vi "MC_10_19a_JW6.vi"() -> ()   [LabVIEW 2011]
uses:
  <vilib>/Utility/file.llb/Read From Spreadsheet File (string).vi
  <vilib>/Utility/inputDevices.llb/keyboardAcquire.vi
  <vilib>/Utility/file.llb/Write To Spreadsheet File (DBL).vi
  <vilib>/Utility/file.llb/Write To Spreadsheet File (string).vi
  <vilib>/regexp/Match Regular Expression.xnode
panel:
  out "Current \nRecord":string[](array[string])
  out "Transformer \nHeaders":string[](array[string])
  out "Current Device ID":string
  out "Column":string
  out "Row":string
  out "Date Recorded":string="Date Recorded"
  out "Concentration Recorded":string
  out "Solvent Recorded":string
  out "Method Recorded":string
  in  "?":T1(tab)
  out "Material Recorded":string
  in  "Treatment Concentration (mM):":dbl=30.0
  in  "Surface Treatment:":string
  in  "# Drops:":dbl=inf
  in  "Solution Temp (C):":dbl=55.0
  in  "Relative Humidity (%):":dbl=nan
  in  "Room Temp (F):":dbl=nan
  in  "Time (s):":dbl=80.0
  out "Accel (RPM/s):":dbl
  in  "RPM:":dbl=1000.0
  in  "Wait Time (s):":dbl=10.0
  in  "Sample #:":dbl=1.0
  in  "Fabricator:":string="Jeremy"
  in  "Data File":path
  out "Data Folder":path
  in  "Image Folder":path
  out "Image File":path
  in  "Ramp (s):":dbl=3.0
  out "Mobility":dbl format="%#_4e"
  out "Length":dbl
  out "Width":dbl
  out "Dielectric (d)":dbl
  out "XY Graph":cluster{dbl[], dbl[]}[](graph)
  in  "NumPts":dbl=5.0
  in  "Cancel Button":bool
  in  "Next Button":bool
  in  "Previous Button":bool
  in  "Up Button":bool
  in  "Down Button":bool
  out "Data Name":string
  in  "Save Changes?":bool
  in  "New Dielectric":dbl
  in  "New Length":dbl
  in  "New Width":dbl
  out "New Mobility":dbl format="%#_4e"
  in  "Slide":dbl(slide) step=1.0 scale=-14.3..84.0 scale format="%#_1p"
  in  "Blank Button":bool
  in  "Zoom":i16(slide)=-3 scale=-5.0..5.0
  out "Image Out 2":T2(plugin-control)
  out "Image Out":T2(plugin-control)
  in  "Magnification":u16(ring) items=["5x", "10x", "20x", "50x", "80x"]
  out "Total Width":dbl
  out "Distances":dbl[](array[numeric])
  in  "Undo Button":bool
  in  "Remove Button":bool
  out "Recorded Mobility":dbl format="%#_4e"
  out "Index 3":string
  out "Image Name":string
  in  "Export":bool
  out "Threshold V":dbl
  out "New Vt":dbl
  in  "Manual":bool
  out "XY Graph 2":cluster{dbl[], dbl[]}[](graph)
  in  "Next Button 2":bool
  in  "Previous Button 2":bool
  in  "Slide 2":dbl(slide) step=1.0 scale=-1.0..82.0 scale format="%#_1p"
  out "S.T.S.":dbl
  out "New S.T.S.":dbl
  in  "NumPts 2":dbl=5.0
  out "Vt recorded":dbl
  out "STS recorded":dbl
  out "On/Off":dbl format="%#_3e"
  in  "Save Changes? 2":bool
  in  "Save Changes? 3":bool
  out "String":string
  in  "No Image":path=path "C:/Program Files/Mega Awesome/Image Not Found.png"
  in  "Project":path=path "C:/Program Files/Mega Awesome/DeviceData.opj"
  out "Index 2":dbl
  out "Array 8":dbl[](array[numeric])
  out "Array 7":dbl[](array[numeric])
  out "ROI Descriptor out":T3 {"Contours"."Type" items=["No Selection", "Point", "Line", "Rectangle", "Oval", "Polygon", "Freehand Region", "Annulus", "Unused2", "Unused3", "Broken Line", "Freehand Line", "Rotated Rectangle"]}
  out "ROI Descriptor":T3 {"Contours"."Type" items=["No Selection", "Point", "Line", "Rectangle", "Oval", "Polygon", "Freehand Region", "Annulus", "Unused2", "Unused3", "Broken Line", "Freehand Line", "Rotated Rectangle"]}
  out "Numeric 3":dbl
  out "Array 6":dbl[][](array[numeric])
  out "Cluster":T4
  out "Array 5":dbl[](array[numeric])
  out "Array 4":dbl[](array[numeric])
  out "Array 3":dbl[](array[numeric])
  out "Numeric 2":dbl
  out "Numeric":dbl
  out "Array 2":dbl[](array[numeric])
  out "Array":dbl[](array[numeric])
  out "Index":dbl
  out "Table Control 2":string[][](table)
  out "Table Control":string[][](table)
  in  "Row Start":dbl=20.0
  # "Data Locations"
  # "Data Location"
  # "Image Location"
  # "Sample Properties"
  # "Recorded"
  # "Calculated"
  # "Re-Calculated"
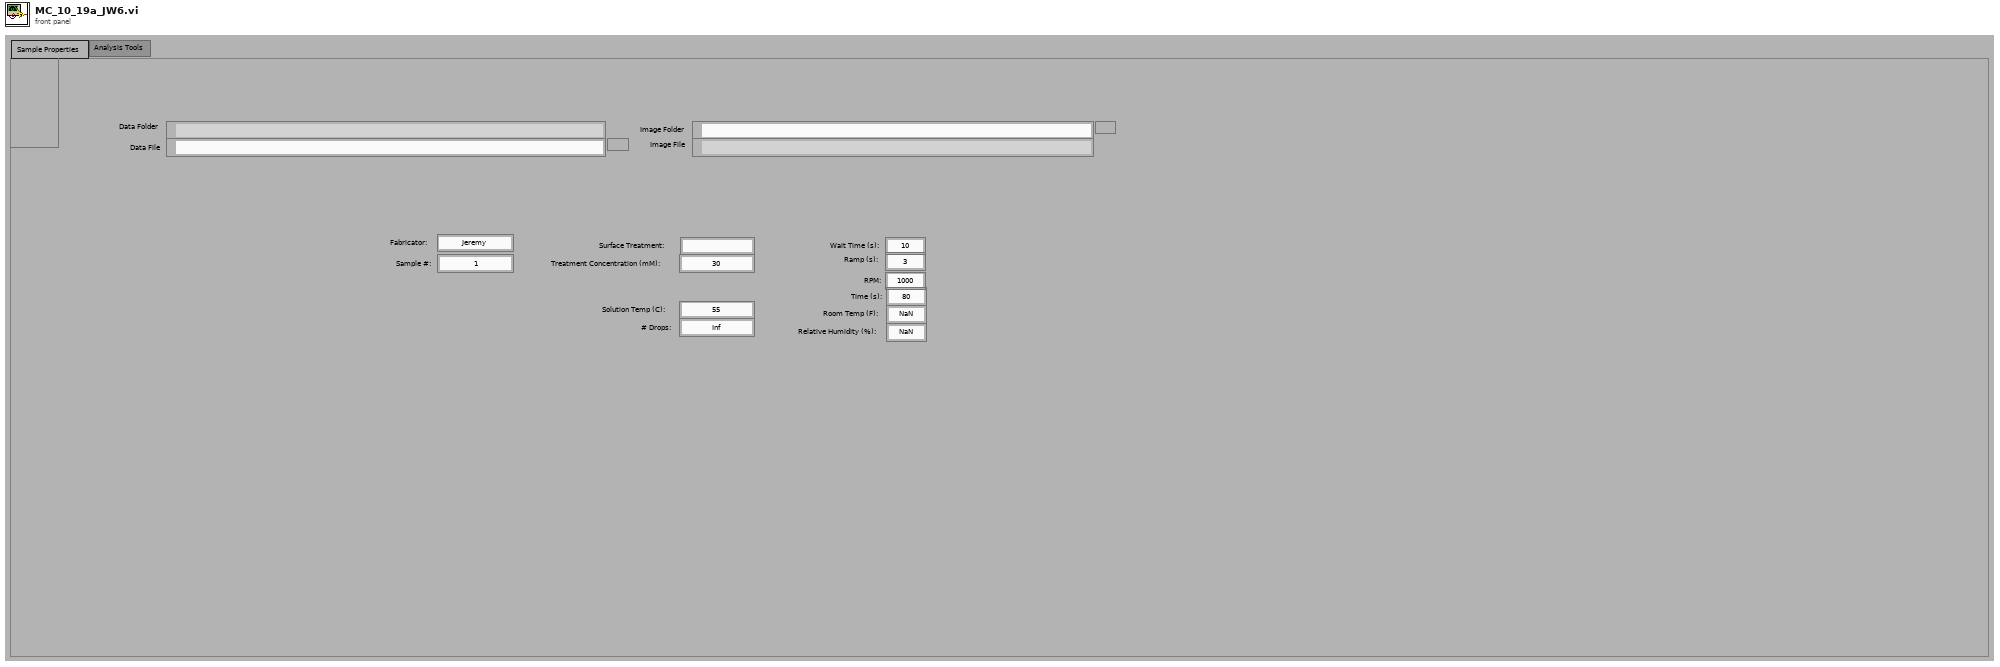
[diagram p1: front panel]
types:
  T1 = enum32{"Sample Properties", "Analysis Tools", "Current Database"}
  T2 = typedef "IMAQ Image.ctl" = refnum<image>
  T3 = typedef "ROI Descriptor" = cluster{"Global Rectangle":i32[], "Contours":cluster{"ID":enum32{"External", "Internal"}, "Type":u32, "Coordinates":i32[]}[]}
  T4 = cluster{"Numeric":dbl, "Numeric 2":dbl, "Numeric 3":dbl, "Numeric 4":dbl}
  T5 = cluster{"[0]":cluster{dbl[], dbl[]}, "[1]":cluster{dbl[], dbl[]}, "[2]":cluster{dbl[], dbl[]}, "[3]":cluster{dbl[], dbl[]}, "[4]":cluster{dbl[], dbl[]}, "[5]":cluster{dbl[], dbl[]}, "[6]":cluster{dbl[], dbl[]}, "[7]":cluster{dbl[], dbl[]}, "[8]":cluster{dbl[], dbl[]}}
  T6 = cluster{"Vt":dbl, "STS":dbl, "On/Off":dbl, "Deposition":string, "Solvent":string, "Concentration":string, "Material":string}
  T7 = cluster{"Global Rectangle":i32[], "Contours":cluster{"Contour Type":u32, "ROI Type":u32, "Points":i32[]}[]}
  T8 = typedef "LVBoundsTypeDef.ctl" = cluster{"Width":u32, "Height":u32}
  T9 = cluster{"Contour Type":u32, "ROI Type":u32, "Points":i32[]}[]
  T10 = enum16{"0", "1", "2", "3", "4", "5", "6", "7", "8", "9", "A", "B", "C", "D", "E", "F", "G", "H", "I", "J", "K", "L", "M", "N", "O", "P", "Q", "R", "S", "T", "U", "V", "W", "X", "Y", "Z", "F1", "F2", "F3", "F4", "F5", "F6", "F7", "F8", "F9", "F10", "F11", "F12", "F13", "F14", "F15", "ADD", "BACK", "BACKSLASH", "CAPITAL", "COMMA", "DECIMAL", "DELETE", "DIVIDE", "DOWN", "END", "EQUALS", "ESCAPE", "GRAVE (`)", "HOME", "INSERT", "LBRACKET", "LCONTROL", "LEFT", "L ALT", "LSHIFT", "LWIN", "MINUS", "MULTIPLY", "NEXT", "NUMLOCK", "NUMPAD_0", "NUMPAD_1", "NUMPAD_2", "NUMPAD_3", "NUMPAD_4", "NUMPAD_5", "NUMPAD_6", "NUMPAD_7", "NUMPAD_8", "NUMPAD_9", "PAUSE", "PERIOD", "PRIOR (PG UP)", "RBRACKET", "RCONTROL", "RETURN", "RIGHT", "R ALT", "RSHIFT", "RWIN", "SCROLL", "SEMICOLON", "SLASH", "SPACE", "SUBTRACT", "TAB", "UP", "ENTER (num pad)", "' (quote)"}[]
  T11 = cluster{i32[], cluster{"Contour Type":u32, "ROI Type":u32, "Points":i32[]}[]}
  T12 = enum16{"0", "1", "2", "3", "4", "5", "6", "7", "8", "9", "A", "B", "C", "D", "E", "F", "G", "H", "I", "J", "K", "L", "M", "N", "O", "P", "Q", "R", "S", "T", "U", "V", "W", "X", "Y", "Z", "F1", "F2", "F3", "F4", "F5", "F6", "F7", "F8", "F9", "F10", "F11", "F12", "F13", "F14", "F15", "ADD", "BACK", "BACKSLASH", "CAPITAL", "COMMA", "DECIMAL", "DELETE", "DIVIDE", "DOWN", "END", "EQUALS", "ESCAPE", "GRAVE (`)", "HOME", "INSERT", "LBRACKET", "LCONTROL", "LEFT", "L ALT", "LSHIFT", "LWIN", "MINUS", "MULTIPLY", "NEXT", "NUMLOCK", "NUMPAD_0", "NUMPAD_1", "NUMPAD_2", "NUMPAD_3", "NUMPAD_4", "NUMPAD_5", "NUMPAD_6", "NUMPAD_7", "NUMPAD_8", "NUMPAD_9", "PAUSE", "PERIOD", "PRIOR (PG UP)", "RBRACKET", "RCONTROL", "RETURN", "RIGHT", "R ALT", "RSHIFT", "RWIN", "SCROLL", "SEMICOLON", "SLASH", "SPACE", "SUBTRACT", "TAB", "UP", "ENTER (num pad)", "' (quote)"}
  T13 = cluster{string, sgl, bool, bool, bool, bool, bool, bool, i32}
  T14 = cluster{i32, cluster{string, sgl, bool, bool, bool, bool, bool, bool, i32}, i32, i32}
  T15 = cluster{"Contour Type":u32, "ROI Type":u32, "Points":i32[]}
  T16 = cluster{"Points[0]":i32, "Points[1]":i32, "Points[2]":i32, "Points[3]":i32, "Points[4]":i32, "Points[5]":i32, "Points[6]":i32, "Points[7]":i32, "Points[8]":i32}
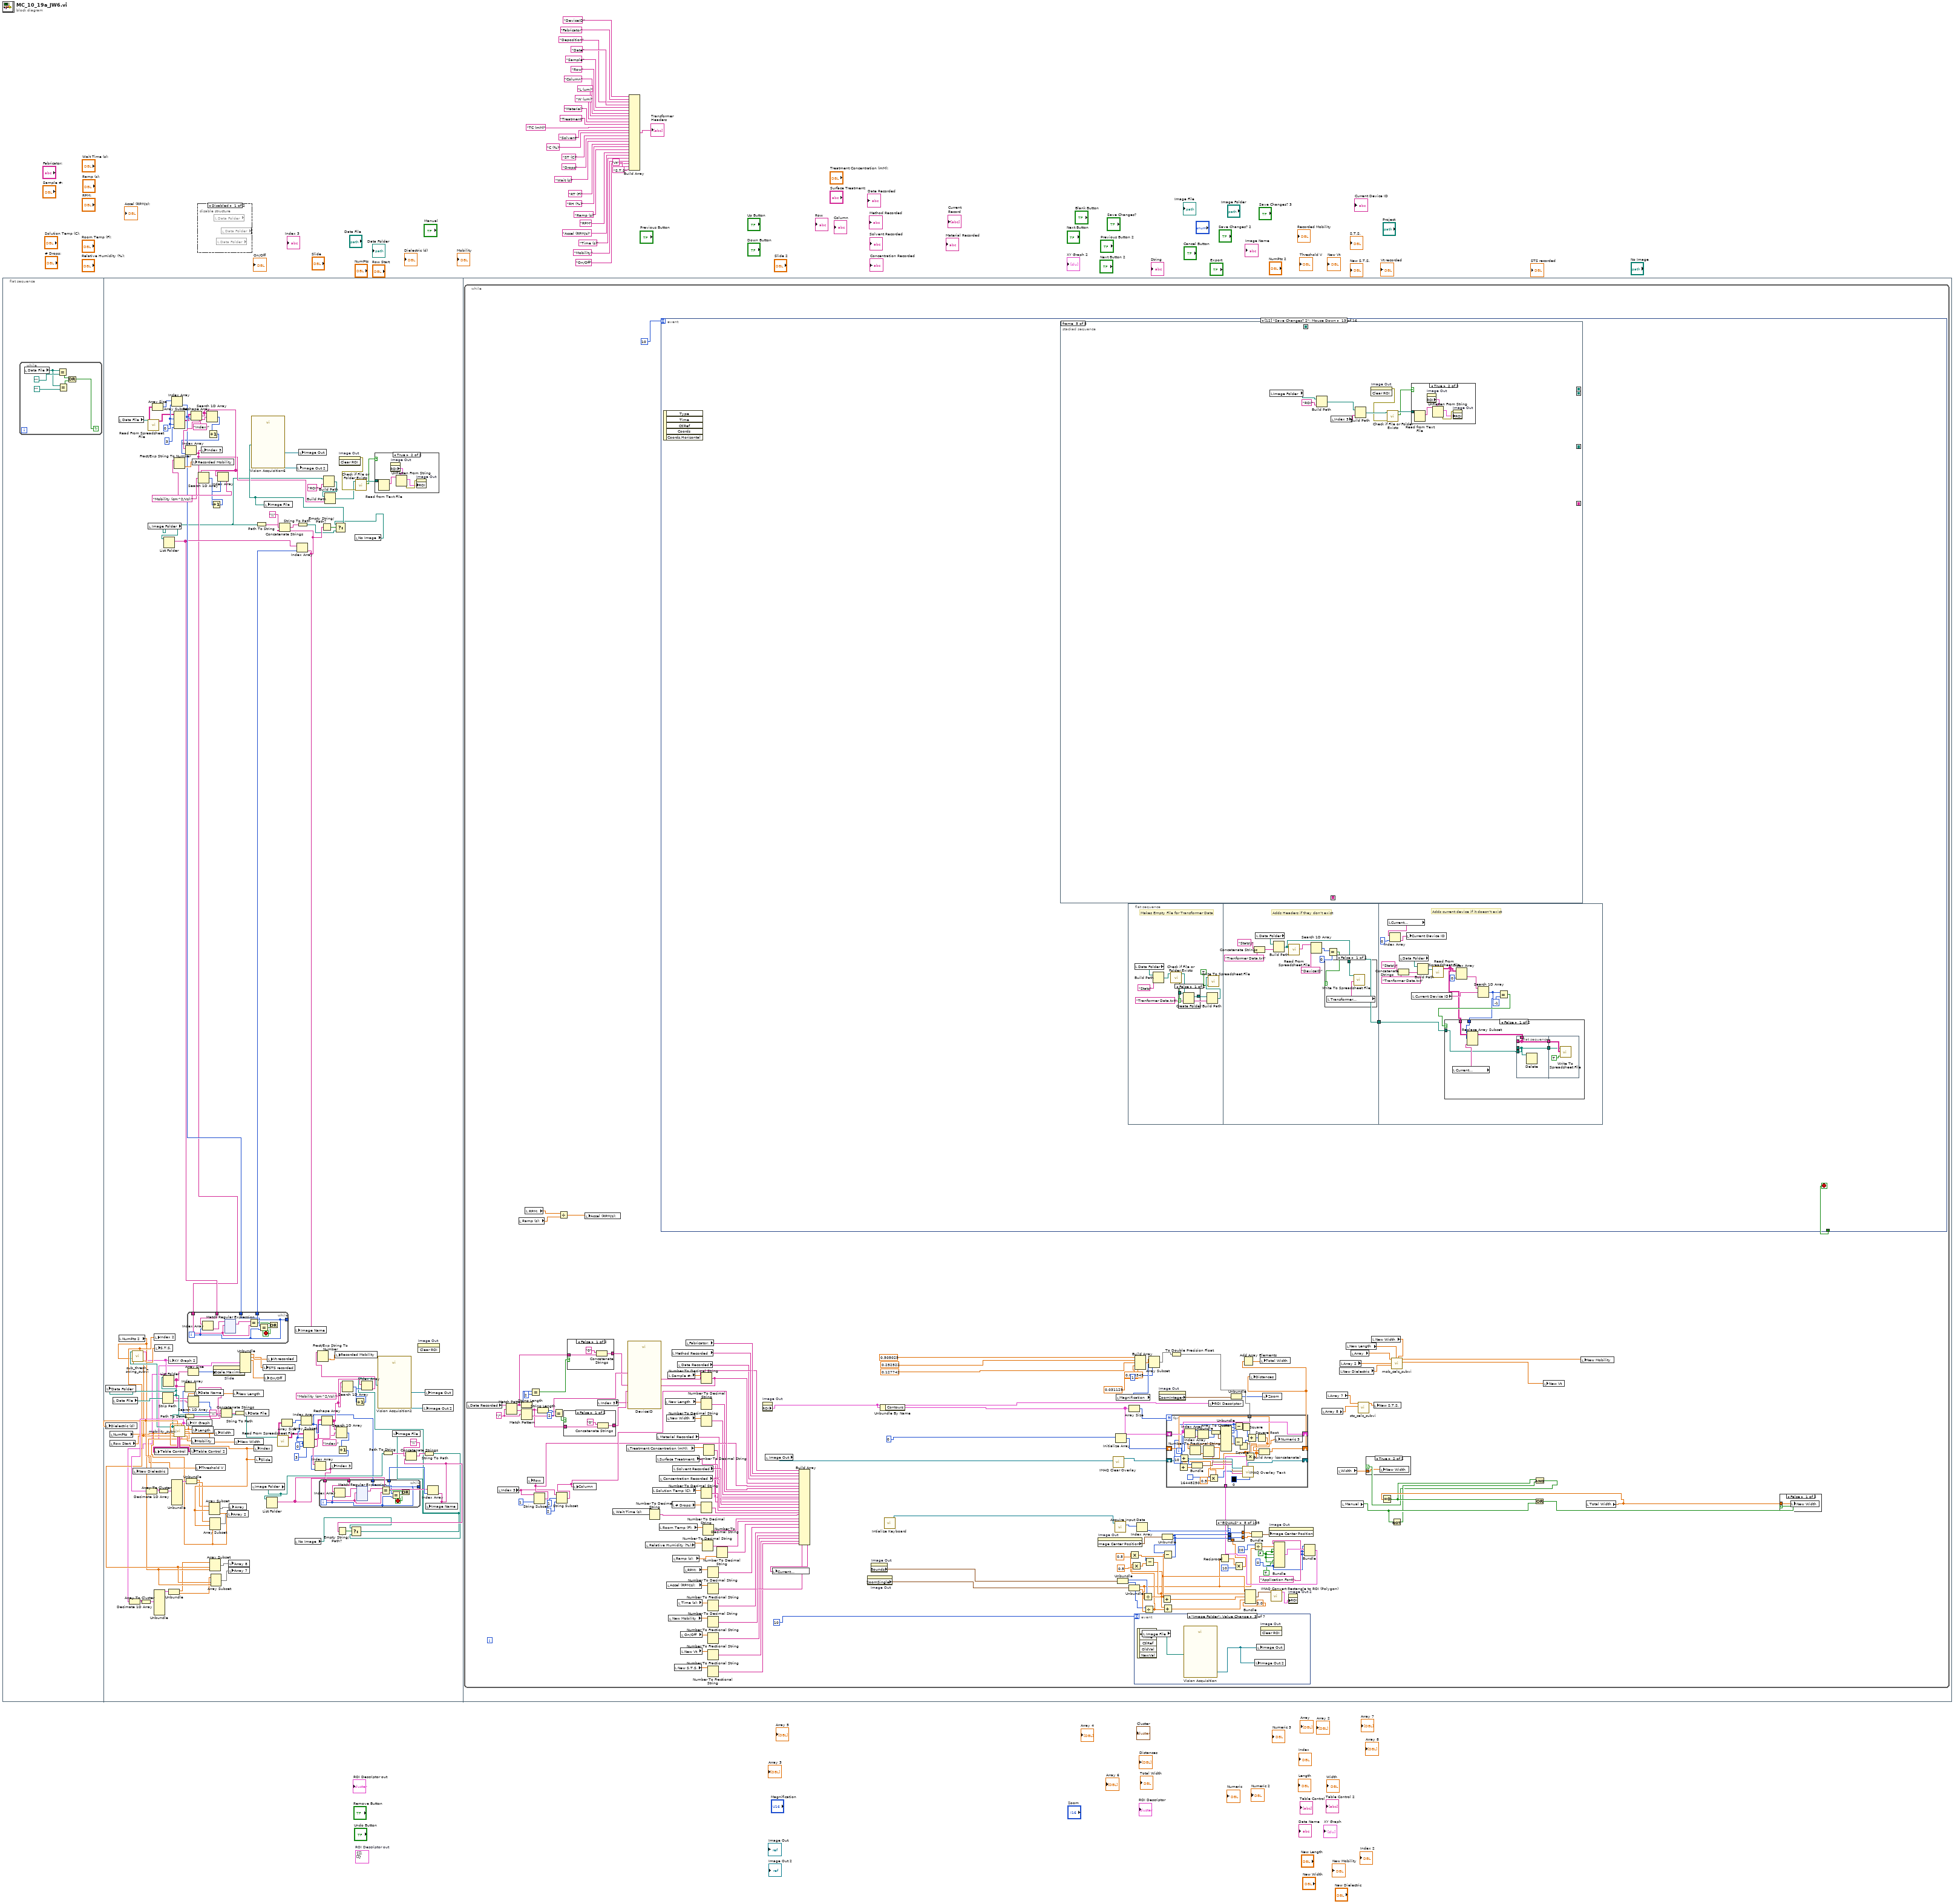
[diagram p0: block diagram]
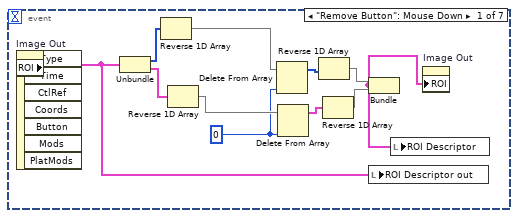
[diagram p7: hidden frame]
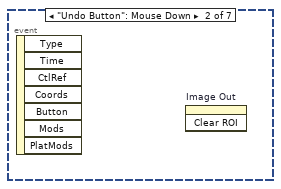
[diagram p8: hidden frame]
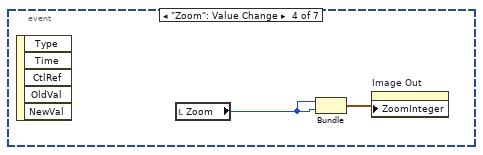
[diagram p9: hidden frame]
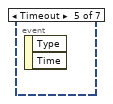
[diagram p10: hidden frame]
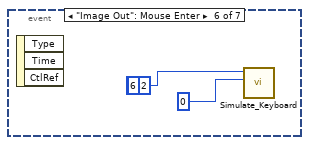
[diagram p11: hidden frame]
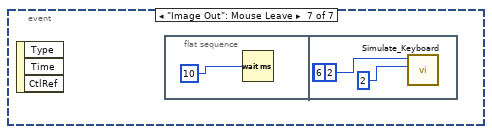
[diagram p12: hidden frame]
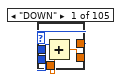
[diagram p13: hidden frame]
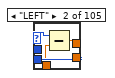
[diagram p14: hidden frame]
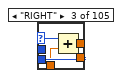
[diagram p15: hidden frame]
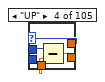
[diagram p16: hidden frame]
diagram:
  (unwired) T3 {"Global Rectangle"=[], "Contours"=[]}  # ROI Descriptor out
  n1 = flat-sequence {
    frame #0 {
      n2 = while {
        stop <- w29 continue-if-true
        n3 = local read "Data File"() -> (w31:path)
        n4 = Equal?(x=w31, y=path "") -> (x = y?=w33:bool)
        n5 = Equal?(x=w31, y=path "") -> (x = y?=w32:bool)
        n6 = Or(x=w33, y=w32) -> (x .or. y?=w29:bool)
      }
    }
    frame #1 {
      w95 = 0
      w125 = 0
      n7 = local read "NumPts"() -> (w70:dbl)
      n8 = local read "Row Start"() -> (w69:dbl)
      n9 = local read "Data File"() -> (w99:path)
      n10 = local read "Data File"() -> (w120:path)
      n11 = local read "NumPts 2"() -> (w64:dbl)
      n12 = call-poly <vilib>:"Read From Spreadsheet File.vi"("file path (dialog if empty)"=w120) -> ("all rows"=w123:string[][])  [unwired: 6 in, 4 out]
      n13 = local read "Image Folder"() -> (w35:path)
      n14 = Array Size(array=w123) -> (size(s)=w124:i32[])
      n15 = Strip Path(path=w99) -> (stripped path=w100:path, name=w81:string)
      n16 = local write "Data Folder"(w100) -> ()
      n17 = List Folder(path=w100) -> (filenames=w89:string[])  [unwired: 3 in, 3 out]
      n18 = List Folder(path=w35) -> (filenames=w129:string[])  [unwired: 3 in, 3 out]
      n19 = Index Array(array=w124, index=w125) -> (element=w131:i32)
      n20 = Array Subset(array=w123, index (row)=w125, index (col)=w125, length (col)=3) -> (w122:string[][])  [unwired: 1 in]
      n21 = Path To String(path=w100) -> (string=w80:string)
      n22 = Array Size(array=w89) -> (size(s)=w90:i32)
      n23 = Search 1D Array(1D array=w89, element=w81) -> (index of element=w88:i32)  [unwired: 1 in]
      n24 = Index Array(array=w89, index=w88) -> (element=w87:string)
      n25 = Reshape Array(w122, w131) -> (w141:string[])
      n26 = local write "Data Name"(w87) -> ()
      n27 = Search 1D Array(1D array=w141, element="Mobility (cm^2/Vs):") -> (index of element=w136:i32)  [unwired: 1 in]
      n28 = Search 1D Array(1D array=w141, element="Index:") -> (index of element=w128:i32)  [unwired: 1 in]
      n29 = Increment(x=w128) -> (x+1=w127:i32)
      n30 = Index Array(array=w141, index=w127) -> (element=w36:string)
      n31 = while {
        tunnel: w129 -> [w274]
        tunnel: w36 -> [w272]
        tunnel: [w271] -> _
        tunnel: [w271] -> w130
        tunnel: w131 -> [w270]
        i -> [w271]
        stop <- w267 stop-if-true
        n32 = Index Array(array=w274, index=w271) -> (element=w275:string)
        n33 = xnode "Match Regular Expression"("input string"=w275, "regular expression"=w272) -> ("whole match"=w273:string)  [unwired: 4 in, 4 out]
        n34 = Equal?(x=w273, y=w272) -> (x = y?=w269:bool)
        n35 = Equal?(x=w270, y=w271) -> (x = y?=w268:bool)
        n36 = Or(x=w269, y=w268) -> (x .or. y?=w267:bool)
      }
      n37 = local write "Index 3"(w36) -> ()
      n38 = Increment(x=w136) -> (x+1=w137:i32)
      n39 = property on="Slide" class="Slide (strict)"("Scale.Maximum"=w90) -> ()  [unwired: 2 in, 2 out]
      n40 = Index Array(array=w141, index=w137) -> (element=w139:string)
      n41 = Fract/Exp String To Number(string=w139) -> (number=w140:dbl)  [unwired: 3 in, 1 out]
      n42 = local write "Recorded Mobility"(w140) -> ()
      n43 = Concatenate Strings(w80, "\\", w87) -> (w82:string)
      n44 = String To Path(string=w82) -> (path=w71:path)
      n45 = call "sub_thresh_swing_subvi.vi"("Path"=w71, "NumPts"=w64, "Row Start"=w69) -> ("Index"=w65:dbl, "XY Graph"=w60:cluster{dbl[], dbl[]}[], "Sub Threshold Swing"=w72:dbl)  [unwired: 8 in, 2 out]
      n46 = Decimate 1D Array(w60) -> (w61:cluster{dbl[], dbl[]}[])  [unwired: 1 out]
      n47 = Array To Cluster(array=w61) -> (cluster=w63:T5)
      n48 = local write "Index 2"(w65) -> ()
      n49 = Unbundle(w63) -> ("[0]"=w62:cluster{dbl[], dbl[]})  [unwired: 8 out]
      n50 = local write "S.T.S."(w72) -> ()
      n51 = local write "XY Graph 2"(w60) -> ()
      n52 = Unbundle(w62) -> (w58:dbl[], w57:dbl[])
      n53 = call "mobility_subvi.vi"("Path"=w71, "NumPts"=w70, "Row Start"=w69) -> ("Dielectric (d)"=w76:dbl, "Index"=w77:dbl, "XY Graph"=w119:cluster{dbl[], dbl[]}[], "Length"=w75:dbl, "Vt"=w73:dbl, "Width"=w74:dbl, "Table Control"=w84:string[][], "Table Control 2"=w85:string[][], "Recorded"=w54:T6, "Mobility"=w86:dbl)  [unwired: 2 in, 1 out]
      n54 = local write "Dielectric (d)"(w76) -> ()
      n55 = local write "New Dielectric"(w76) -> ()
      n56 = Decimate 1D Array(w119) -> (w118:cluster{dbl[], dbl[]}[])  [unwired: 1 out]
      n57 = local write "Table Control"(w84) -> ()
      n58 = Array To Cluster(array=w118) -> (cluster=w116:T5)
      n59 = Unbundle(w116) -> ("[0]"=w117:cluster{dbl[], dbl[]})  [unwired: 8 out]
      n60 = Unbundle(w117) -> (w59:dbl[], w66:dbl[])
      n61 = local write "XY Graph"(w119) -> ()
      n62 = local write "Table Control 2"(w85) -> ()
      n63 = local write "Mobility"(w86) -> ()
      n64 = local write "Length"(w75) -> ()
      n65 = local write "Threshold V"(w73) -> ()
      n66 = Array Subset(array=w59, index=w77, length=w70) -> (w78:dbl[])
      n67 = Array Subset(array=w66, index=w77, length=w70) -> (w79:dbl[])
      n68 = Array Subset(array=w58, index=w65, length=w64) -> (w68:dbl[])
      n69 = Array Subset(array=w57, index=w65, length=w64) -> (w67:dbl[])
      n70 = local write "Width"(w74) -> ()
      n71 = local write "Array 2"(w79) -> ()
      n72 = local write "Array 8"(w68) -> ()
      n73 = local write "Array 7"(w67) -> ()
      n74 = local write "Array"(w78) -> ()
      n75 = local write "New Length"(w75) -> ()
      n76 = local write "New Width"(w74) -> ()
      n77 = Unbundle(w54) -> ("Vt"=w56:dbl, "STS"=w55:dbl, "On/Off"=w53:dbl)  [unwired: 4 out]
      n78 = local write "Data File"(w71) -> ()
      n79 = local read "Image Folder"() -> (w106:path)
      n80 = local write "Index"(w77) -> ()
      n81 = local write "Slide"(w77) -> ()
      n82 = Path To String(path=w35) -> (string=w133:string)
      n83 = local write "STS recorded"(w55) -> ()
      n84 = local write "On/Off"(w53) -> ()
      n85 = List Folder(path=w106) -> (filenames=w102:string[])  [unwired: 3 in, 3 out]
      n86 = local write "Vt recorded"(w56) -> ()
      n87 = call-poly <vilib>:"Read From Spreadsheet File.vi"("file path (dialog if empty)"=w71) -> ("all rows"=w93:string[][])  [unwired: 6 in, 4 out]
      n88 = Array Size(array=w93) -> (size(s)=w94:i32[])
      n89 = local read "No Image"() -> (w44:path)
      n90 = Index Array(array=w129, index=w130) -> (element=w52:string)
      n91 = Concatenate Strings(w133, "\\", w52) -> (w134:string)
      n92 = local write "Image Name"(w52) -> ()
      n93 = String To Path(string=w134) -> (path=w50:path)
      n94 = Index Array(array=w94, index=w95) -> (element=w105:i32)
      n95 = Array Subset(array=w93, index (row)=w95, index (col)=w95, length (col)=3) -> (w92:string[][])  [unwired: 1 in]
      n96 = Empty String/Path?(string/path=w52) -> (empty?=w51:bool)
      n97 = Reshape Array(w92, w105) -> (w115:string[])
      n98 = Build Path(base path=w35, name or relative path="ROI") -> (appended path=w38:path)
      n99 = Build Path(base path=w38, name or relative path=w36) -> (appended path=w37:path)
      n100 = Search 1D Array(1D array=w115, element="Index:") -> (index of element=w98:i32)  [unwired: 1 in]
      n101 = Increment(x=w98) -> (x+1=w97:i32)
      n102 = Index Array(array=w115, index=w97) -> (element=w103:string)
      n103 = while {
        tunnel: w102 -> [w154]
        tunnel: w103 -> [w152]
        tunnel: [w151] -> _
        tunnel: [w151] -> w104
        tunnel: w105 -> [w150]
        i -> [w151]
        stop <- w147 stop-if-true
        n104 = Index Array(array=w154, index=w151) -> (element=w155:string)
        n105 = xnode "Match Regular Expression"("input string"=w155, "regular expression"=w152) -> ("whole match"=w153:string)  [unwired: 4 in, 4 out]
        n106 = Equal?(x=w153, y=w152) -> (x = y?=w149:bool)
        n107 = Equal?(x=w150, y=w151) -> (x = y?=w148:bool)
        n108 = Or(x=w149, y=w148) -> (x .or. y?=w147:bool)
      }
      n109 = local write "Index 3"(w103) -> ()
      n110 = invoke on="Image Out" class="ImageControl" method="Clear ROI"() -> (error out=w42:errorcluster)  [unwired: 3 in, 2 out]
      n111 = Search 1D Array(1D array=w115, element="Mobility (cm^2/Vs):") -> (index of element=w110:i32)  [unwired: 1 in]
      n112 = local read "No Image"() -> (w43:path)
      n113 = Select(t=w43, s=w51, f=w50) -> (s? t:f=w49:path)
      n114 = call "Vision Acquisition6"("Image Path"=w49) -> ("Image Out"=w132:T2)  [unwired: 25 in, 1 out]
      n115 = local write "Image File"(w49) -> ()
      n116 = local write "Image Out 2"(w132) -> ()
      n117 = local write "Image Out"(w132) -> ()
      n118 = Increment(x=w110) -> (x+1=w111:i32)
      n119 = call <vilib>:"Check if File or Folder Exists.vi"("error in (no error)"=w42, "path"=w37) -> ("file or folder exists?"=w40:bool, "dup path"=w41:path)  [unwired: 7 in, 1 out]
      n120 = Index Array(array=w115, index=w111) -> (element=w113:string)
      n121 = Fract/Exp String To Number(string=w113) -> (number=w114:dbl)  [unwired: 3 in, 1 out]
      n122 = local write "Recorded Mobility"(w114) -> ()
      n123 = case shown="True" w40 {
        tunnel: w41 -> [_ w142]
        frame False {
        }
        frame True {
          n124 = Read from Text File(file (use dialog)=w142) -> (text=w146:string)  [unwired: 3 in, 3 out]
          n125 = property on="Image Out" class="ImageControl"() -> ("ROI"=w143:T7)  [unwired: 2 in, 2 out]
          n126 = Unflatten From String(type=w143, binary string=w146) -> (value=w144:T7, error out=w145:errorcluster)  [unwired: 3 in, 1 out]
          n127 = property on="Image Out" class="ImageControl"(error in=w145, "ROI"=w144) -> ()  [unwired: 1 in, 2 out]
        }
      }
      n128 = Path To String(path=w106) -> (string=w107:string)
      n129 = invoke on="Image Out" class="ImageControl" method="Clear ROI"() -> ()  [unwired: 3 in, 3 out]
      n130 = Index Array(array=w102, index=w104) -> (element=w47:string)
      n131 = Empty String/Path?(string/path=w47) -> (empty?=w48:bool)
      n132 = Concatenate Strings(w107, "\\", w47) -> (w108:string)
      n133 = String To Path(string=w108) -> (path=w46:path)
      n134 = Select(t=w44, s=w48, f=w46) -> (s? t:f=w45:path)
      n135 = call "Vision Acquisition2"("Image Path"=w45) -> ("Image Out"=w101:T2)  [unwired: 25 in, 1 out]
      n136 = local write "Image File"(w45) -> ()
      n137 = local write "Image Out 2"(w101) -> ()
      n138 = local write "Image Out"(w101) -> ()
      n139 = local write "Image Name"(w47) -> ()
    }
    frame #2 {
      n140 = while {
        stop <- w533 stop-if-true
        w419 = "/"
        w483 = FALSE
        w481 = 0
        n141 = local read "Date Recorded"() -> (w422:string)
        n142 = local read "Index 3"() -> (w391:string)
        n143 = Match Pattern(string=w422, regular expression=w419) -> (before substring=w413:string, after substring=w420:string)  [unwired: 1 in, 2 out]
        n144 = local read "Ramp (s):"() -> (w388:dbl)
        n145 = String Length(string=w413) -> (length=w416:i32)
        n146 = Match Pattern(string=w420, regular expression=w419) -> (before substring=w407:string, after substring=w418:string)  [unwired: 1 in, 2 out]
        n147 = local read "RPM:"() -> (w389:dbl)
        n148 = Equal?(x=w416, y=2) -> (x = y?=w414:bool)
        n149 = String Subset(string=w391, length (rest)=1) -> (substring=w447:string)  [unwired: 1 in]
        n150 = local write "Row"(w447) -> ()
        n151 = String Length(string=w407) -> (length=w409:i32)
        n152 = Equal?(x=w409, y=2) -> (x = y?=w411:bool)
        n153 = String Subset(string=w391, offset (0)=1, length (rest)=2) -> (substring=w448:string)
        n154 = Divide(x=w389, y=w388) -> (x/y=w387:dbl)
        n155 = case shown="False" w411 {
          tunnel: w407 -> [w535 w537]
          tunnel: [w534 w537] -> w408
          frame False {
            n156 = Concatenate Strings("0", w535) -> (w534:string)
          }
          frame True {
          }
        }
        n157 = case shown="False" w414 {
          tunnel: w413 -> [w539 w541]
          tunnel: [w538 w541] -> w412
          frame False {
            n158 = Concatenate Strings("0", w539) -> (w538:string)
          }
          frame True {
          }
        }
        n159 = local write "Column"(w448) -> ()
        n160 = local write "Accel (RPM/s):"(w387) -> ()
        n161 = local read "Index 3"() -> (w406:string)
        n162 = local read "Wait Time (s):"() -> (w452:dbl)
        n163 = local read "Treatment Concentration (mM):"() -> (w399:dbl)
        n164 = local read "Relative Humidity (%):"() -> (w396:dbl)
        n165 = Number To Decimal String(number=w452) -> (decimal integer string=w453:string)  [unwired: 1 in]
        n166 = local read "Solution Temp (C):"() -> (w441:dbl)
        n167 = local read "Surface Treatment:"() -> (w398:string)
        n168 = local read "Material Recorded"() -> (w394:string)
        n169 = local read "Room Temp (F):"() -> (w445:dbl)
        n170 = local read "Concentration Recorded"() -> (w401:string)
        n171 = event shown="[12] \"Save Changes? 2\": Mouse Down" {
          selector: _ -> [_ _ _ _ _ _ _ _ _ _ _ _ _ _ _ _]
          dyn-events: _ -> [_ _ _ _ _ _ _ _ _ _ _ _ _ _ _ _]
          timeout: 10 -> [_ _ _ _ _ _ _ _ _ _ _ _ _ _ _ _]
          tunnel: [_ _ _ _ _ _ _ _ _ _ _ _ _ TRUE _ TRUE] -> w533
          event Timeout {
            n172 = event-data() -> ()  [unwired: 1 in, 2 out]
          }
          event "Down Button": Mouse Down {
            w889 = 0
            n173 = event-data() -> ()  [unwired: 1 in, 7 out]
            n174 = local read "NumPts 2"() -> (w850:dbl)
            n175 = local read "NumPts"() -> (w857:dbl)
            n176 = local read "Row Start"() -> (w856:dbl)
            n177 = local read "Data File"() -> (w894:path)
            n178 = property on="Image Out" class="ImageControl"() -> (error out=w819:errorcluster, "Image Center Position"=w823:cluster{"X":u32, "Y":u32})  [unwired: 2 in, 1 out]
            n179 = Unbundle(w823) -> ("X"=w821:u32)  [unwired: 1 out]
            n180 = Strip Path(path=w894) -> (stripped path=w885:path, name=w907:string)
            n181 = local write "Data Folder"(w885) -> ()
            n182 = List Folder(path=w885) -> (filenames=w900:string[], error out=w828:errorcluster)  [unwired: 3 in, 2 out]
            n183 = Array Size(array=w900) -> (size(s)=w895:i32)
            n184 = Bundle("X"=w821, 0) -> (w822:cluster{"X":u32, i32})  [unwired: 1 in]
            n185 = Path To String(path=w885) -> (string=w908:string)
            n186 = Search 1D Array(1D array=w900, element=w907) -> (index of element=w897:i32)  [unwired: 1 in]
            n187 = property on="Image Out" class="ImageControl"(error in=w819, "Image Center Position"=w822) -> ()  [unwired: 1 in, 2 out]
            n188 = Decrement(x=w895) -> (x-1=w898:i32)
            n189 = Equal?(x=w897, y=w898) -> (x = y?=w899:bool)
            n190 = case shown="False" w899 {
              tunnel: w897 -> [w1035 _]
              tunnel: [w1034 0] -> w896
              frame False {
                n191 = Increment(x=w1035) -> (x+1=w1034:i32)
              }
              frame True {
              }
            }
            n192 = Index Array(array=w900, index=w896) -> (element=w901:string)
            n193 = local write "Data Name"(w901) -> ()
            n194 = Concatenate Strings(w908, "\\", w901) -> (w906:string)
            n195 = String To Path(string=w906) -> (path=w858:path)
            n196 = call "sub_thresh_swing_subvi.vi"("Path"=w858, "NumPts"=w850, "Row Start"=w856) -> ("Index"=w851:dbl, "XY Graph"=w846:cluster{dbl[], dbl[]}[], "Sub Threshold Swing"=w859:dbl)  [unwired: 8 in, 2 out]
            n197 = Decimate 1D Array(w846) -> (w849:cluster{dbl[], dbl[]}[])  [unwired: 1 out]
            n198 = Array To Cluster(array=w849) -> (cluster=w847:T5)
            n199 = Unbundle(w847) -> ("[0]"=w848:cluster{dbl[], dbl[]})  [unwired: 8 out]
            n200 = Unbundle(w848) -> (w845:dbl[], w844:dbl[])
            n201 = local write "S.T.S."(w859) -> ()
            n202 = local write "XY Graph 2"(w846) -> ()
            n203 = local write "Index 2"(w851) -> ()
            n204 = call "mobility_subvi.vi"("Path"=w858, "NumPts"=w857, "Row Start"=w856) -> ("Dielectric (d)"=w861:dbl, "Date Created"=w818:string, "Index"=w866:dbl, "XY Graph"=w869:cluster{dbl[], dbl[]}[], "Length"=w860:dbl, "Vt"=w862:dbl, "Width"=w834:dbl, "Table Control"=w904:string[][], "Table Control 2"=w903:string[][], "Recorded"=w843:T6, "Mobility"=w902:dbl)  [unwired: 2 in]
            n205 = local write "Dielectric (d)"(w861) -> ()
            n206 = local write "Threshold V"(w862) -> ()
            n207 = local write "New Dielectric"(w861) -> ()
            n208 = Decimate 1D Array(w869) -> (w870:cluster{dbl[], dbl[]}[])  [unwired: 1 out]
            n209 = Array To Cluster(array=w870) -> (cluster=w872:T5)
            n210 = local write "Table Control"(w904) -> ()
            n211 = Unbundle(w872) -> ("[0]"=w871:cluster{dbl[], dbl[]})  [unwired: 8 out]
            n212 = Unbundle(w871) -> (w853:dbl[], w852:dbl[])
            n213 = local write "XY Graph"(w869) -> ()
            n214 = local write "Table Control 2"(w903) -> ()
            n215 = local write "Mobility"(w902) -> ()
            n216 = Array Subset(array=w853, index=w866, length=w857) -> (w868:dbl[])
            n217 = Array Subset(array=w852, index=w866, length=w857) -> (w867:dbl[])
            n218 = Unbundle(w843) -> ("Vt"=w842:dbl, "STS"=w841:dbl, "On/Off"=w840:dbl, "Deposition"=w817:string, "Solvent"=w816:string, "Concentration"=w815:string, "Material"=w814:string)
            n219 = local write "On/Off"(w840) -> ()
            n220 = local write "Width"(w834) -> ()
            n221 = local write "Length"(w860) -> ()
            n222 = local write "Array 2"(w867) -> ()
            n223 = local write "Array"(w868) -> ()
            n224 = local write "Slide"(w866) -> ()
            n225 = local write "Index"(w866) -> ()
            n226 = local write "STS recorded"(w841) -> ()
            n227 = local write "Date Recorded"(w818) -> ()
            n228 = local write "Solvent Recorded"(w816) -> ()
            n229 = local write "Concentration Recorded"(w815) -> ()
            n230 = local write "Method Recorded"(w817) -> ()
            n231 = local write "Vt recorded"(w842) -> ()
            n232 = Array Subset(array=w845, index=w851, length=w850) -> (w855:dbl[])
            n233 = Array Subset(array=w844, index=w851, length=w850) -> (w854:dbl[])
            n234 = local write "Material Recorded"(w814) -> ()
            n235 = local write "New Width"(w834) -> ()
            n236 = local write "Data File"(w858) -> ()
            n237 = local write "New Length"(w860) -> ()
            n238 = local write "Array 8"(w855) -> ()
            n239 = local write "Array 7"(w854) -> ()
            n240 = call-poly <vilib>:"Read From Spreadsheet File.vi"("file path (dialog if empty)"=w858) -> ("all rows"=w891:string[][])  [unwired: 6 in, 4 out]
            n241 = local read "Image Folder"() -> (w825:path)
            n242 = Array Size(array=w891) -> (size(s)=w890:i32[])
            n243 = List Folder(path=w825, error in=w828) -> (filenames=w884:string[], error out=w829:errorcluster)  [unwired: 2 in, 2 out]
            n244 = Index Array(array=w890, index=w889) -> (element=w864:i32)
            n245 = Subtract(x=w864, y=20) -> (x-y=w863:i32)
            n246 = property on="Slide" class="Slide (strict)"("Scale.Maximum"=w863) -> ()  [unwired: 2 in, 2 out]
            n247 = Array Subset(array=w891, index (row)=w889, index (col)=w889, length (col)=3) -> (w892:string[][])  [unwired: 1 in]
            n248 = Reshape Array(w892, w864) -> (w873:string[])
            n249 = local read "No Image"() -> (w835:path)
            n250 = Search 1D Array(1D array=w873, element="Mobility (cm^2/Vs):") -> (index of element=w878:i32)  [unwired: 1 in]
            n251 = Search 1D Array(1D array=w873, element="Index:") -> (index of element=w886:i32)  [unwired: 1 in]
            n252 = Increment(x=w886) -> (x+1=w887:i32)
            n253 = Index Array(array=w873, index=w887) -> (element=w827:string)
            n254 = while {
              tunnel: w884 -> [w921]
              tunnel: w827 -> [w919]
              tunnel: [w918] -> _
              tunnel: [w918] -> w883
              tunnel: w864 -> [w917]
              i -> [w918]
              stop <- w914 stop-if-true
              n255 = Index Array(array=w921, index=w918) -> (element=w922:string)
              n256 = xnode "Match Regular Expression"("input string"=w922, "regular expression"=w919) -> ("whole match"=w920:string)  [unwired: 4 in, 4 out]
              n257 = Equal?(x=w920, y=w919) -> (x = y?=w916:bool)
              n258 = Equal?(x=w917, y=w918) -> (x = y?=w915:bool)
              n259 = Or(x=w916, y=w915) -> (x .or. y?=w914:bool)
            }
            n260 = local write "Index 3"(w827) -> ()
            n261 = Increment(x=w878) -> (x+1=w877:i32)
            n262 = Build Path(base path=w825, name or relative path="ROI") -> (appended path=w824:path)
            n263 = Index Array(array=w873, index=w877) -> (element=w875:string)
            n264 = Fract/Exp String To Number(string=w875) -> (number=w874:dbl)  [unwired: 3 in, 1 out]
            n265 = local write "Recorded Mobility"(w874) -> ()
            n266 = Build Path(base path=w824, name or relative path=w827) -> (appended path=w833:path)
            n267 = Path To String(path=w825) -> (string=w881:string)
            n268 = invoke on="Image Out" class="ImageControl" method="Clear ROI"(error in=w829) -> (error out=w832:errorcluster)  [unwired: 2 in, 2 out]
            n269 = call <vilib>:"Check if File or Folder Exists.vi"("error in (no error)"=w832, "path"=w833) -> ("file or folder exists?"=w830:bool, "dup path"=w831:path)  [unwired: 7 in, 1 out]
            n270 = Index Array(array=w884, index=w883) -> (element=w838:string)
            n271 = Empty String/Path?(string/path=w838) -> (empty?=w839:bool)
            n272 = Concatenate Strings(w881, "\\", w838) -> (w880:string)
            n273 = String To Path(string=w880) -> (path=w837:path)
            n274 = Select(t=w835, s=w839, f=w837) -> (s? t:f=w836:path)
            n275 = call "Vision Acquisition4"("Image Path"=w836) -> ("Image Out"=w882:T2)  [unwired: 25 in, 1 out]
            n276 = local write "Image File"(w836) -> ()
            n277 = local write "Image Name"(w838) -> ()
            n278 = local write "Image Out 2"(w882) -> ()
            n279 = local write "Image Out"(w882) -> ()
            n280 = invoke on="Image Out" class="ImageControl" method="Clear ROI"() -> ()  [unwired: 3 in, 3 out]
            n281 = case shown="True" w830 {
              tunnel: w831 -> [_ w909]
              frame False {
              }
              frame True {
                n282 = Read from Text File(file (use dialog)=w909) -> (text=w913:string)  [unwired: 3 in, 3 out]
                n283 = property on="Image Out" class="ImageControl"() -> ("ROI"=w910:T7)  [unwired: 2 in, 2 out]
                n284 = Unflatten From String(type=w910, binary string=w913) -> (value=w911:T7, error out=w912:errorcluster)  [unwired: 3 in, 1 out]
                n285 = property on="Image Out" class="ImageControl"(error in=w912, "ROI"=w911) -> ()  [unwired: 1 in, 2 out]
              }
            }
          }
          event "Data File": Value Change {
            w1108 = 0
            n286 = event-data() -> ()  [unwired: 1 in, 5 out]
            n287 = local read "NumPts"() -> (w1076:dbl)
            n288 = local read "Row Start"() -> (w1075:dbl)
            n289 = local read "Data File"() -> (w1104:path)
            n290 = local read "NumPts 2"() -> (w1069:dbl)
            n291 = property on="Image Out" class="ImageControl"() -> (error out=w1037:errorcluster, "Image Center Position"=w1041:cluster{"X":u32, "Y":u32})  [unwired: 2 in, 1 out]
            n292 = Strip Path(path=w1104) -> (stripped path=w1103:path, name=w1121:string)
            n293 = local write "Data Folder"(w1103) -> ()
            n294 = List Folder(path=w1103) -> (filenames=w1113:string[], error out=w1047:errorcluster)  [unwired: 3 in, 2 out]
            n295 = Unbundle(w1041) -> ("X"=w1039:u32)  [unwired: 1 out]
            n296 = Path To String(path=w1103) -> (string=w1122:string)
            n297 = Search 1D Array(1D array=w1113, element=w1121) -> (index of element=w1114:i32)  [unwired: 1 in]
            n298 = Index Array(array=w1113, index=w1114) -> (element=w1115:string)
            n299 = Bundle("X"=w1039, 0) -> (w1040:cluster{"X":u32, i32})  [unwired: 1 in]
            n300 = local write "Data Name"(w1115) -> ()
            n301 = property on="Image Out" class="ImageControl"(error in=w1037, "Image Center Position"=w1040) -> ()  [unwired: 1 in, 2 out]
            n302 = Concatenate Strings(w1122, "\\", w1115) -> (w1120:string)
            n303 = String To Path(string=w1120) -> (path=w1077:path)
            n304 = call "sub_thresh_swing_subvi.vi"("Path"=w1077, "NumPts"=w1069, "Row Start"=w1075) -> ("Index"=w1070:dbl, "XY Graph"=w1065:cluster{dbl[], dbl[]}[], "Sub Threshold Swing"=w1074:dbl)  [unwired: 8 in, 2 out]
            n305 = Decimate 1D Array(w1065) -> (w1068:cluster{dbl[], dbl[]}[])  [unwired: 1 out]
            n306 = Array To Cluster(array=w1068) -> (cluster=w1066:T5)
            n307 = Unbundle(w1066) -> ("[0]"=w1067:cluster{dbl[], dbl[]})  [unwired: 8 out]
            n308 = Unbundle(w1067) -> (w1063:dbl[], w1062:dbl[])
            n309 = local write "Index 2"(w1070) -> ()
            n310 = call "mobility_subvi.vi"("Path"=w1077, "NumPts"=w1076, "Row Start"=w1075) -> ("Dielectric (d)"=w1079:dbl, "Index"=w1084:dbl, "XY Graph"=w1087:cluster{dbl[], dbl[]}[], "Length"=w1078:dbl, "Vt"=w1080:dbl, "Width"=w1052:dbl, "Table Control"=w1118:string[][], "Table Control 2"=w1117:string[][], "Recorded"=w1059:T6, "Mobility"=w1116:dbl)  [unwired: 2 in, 1 out]
            n311 = local write "Dielectric (d)"(w1079) -> ()
            n312 = local write "New Dielectric"(w1079) -> ()
            n313 = Decimate 1D Array(w1087) -> (w1088:cluster{dbl[], dbl[]}[])  [unwired: 1 out]
            n314 = local write "Table Control"(w1118) -> ()
            n315 = Array To Cluster(array=w1088) -> (cluster=w1090:T5)
            n316 = Unbundle(w1090) -> ("[0]"=w1089:cluster{dbl[], dbl[]})  [unwired: 8 out]
            n317 = local write "Threshold V"(w1080) -> ()
            n318 = local write "S.T.S."(w1074) -> ()
            n319 = Unbundle(w1089) -> (w1064:dbl[], w1071:dbl[])
            n320 = local write "XY Graph"(w1087) -> ()
            n321 = local write "Table Control 2"(w1117) -> ()
            n322 = local write "Mobility"(w1116) -> ()
            n323 = local write "Length"(w1078) -> ()
            n324 = local write "XY Graph 2"(w1065) -> ()
            n325 = Unbundle(w1059) -> ("Vt"=w1061:dbl, "STS"=w1060:dbl, "On/Off"=w1058:dbl)  [unwired: 4 out]
            n326 = local write "On/Off"(w1058) -> ()
            n327 = Array Subset(array=w1063, index=w1070, length=w1069) -> (w1073:dbl[])
            n328 = Array Subset(array=w1062, index=w1070, length=w1069) -> (w1072:dbl[])
            n329 = local write "Width"(w1052) -> ()
            n330 = Array Subset(array=w1064, index=w1084, length=w1076) -> (w1086:dbl[])
            n331 = Array Subset(array=w1071, index=w1084, length=w1076) -> (w1085:dbl[])
            n332 = local write "Array 8"(w1073) -> ()
            n333 = local write "Array 7"(w1072) -> ()
            n334 = local write "STS recorded"(w1060) -> ()
            n335 = local write "Vt recorded"(w1061) -> ()
            n336 = local write "New Length"(w1078) -> ()
            n337 = local write "New Width"(w1052) -> ()
            n338 = local write "Array 2"(w1085) -> ()
            n339 = local write "Array"(w1086) -> ()
            n340 = local write "Data File"(w1077) -> ()
            n341 = local read "Image Folder"() -> (w1043:path)
            n342 = local write "Index"(w1084) -> ()
            n343 = local write "Slide"(w1084) -> ()
            n344 = List Folder(path=w1043, error in=w1047) -> (filenames=w1101:string[], error out=w1046:errorcluster)  [unwired: 2 in, 2 out]
            n345 = call-poly <vilib>:"Read From Spreadsheet File.vi"("file path (dialog if empty)"=w1077) -> ("all rows"=w1110:string[][])  [unwired: 6 in, 4 out]
            n346 = Array Size(array=w1110) -> (size(s)=w1109:i32[])
            n347 = Index Array(array=w1109, index=w1108) -> (element=w1083:i32)
            n348 = Subtract(x=w1083, y=20) -> (x-y=w1081:i32)
            n349 = property on="Slide" class="Slide (strict)"("Scale.Maximum"=w1081) -> ()  [unwired: 2 in, 2 out]
            n350 = Array Subset(array=w1110, index (row)=w1108, index (col)=w1108, length (col)=3) -> (w1111:string[][])  [unwired: 1 in]
            n351 = Reshape Array(w1111, w1083) -> (w1091:string[])
            n352 = Search 1D Array(1D array=w1091, element="Index:") -> (index of element=w1105:i32)  [unwired: 1 in]
            n353 = Increment(x=w1105) -> (x+1=w1106:i32)
            n354 = Index Array(array=w1091, index=w1106) -> (element=w1045:string)
            n355 = while {
              tunnel: w1101 -> [w1135]
              tunnel: w1045 -> [w1133]
              tunnel: [w1132] -> _
              tunnel: [w1132] -> w1100
              tunnel: w1083 -> [w1131]
              i -> [w1132]
              stop <- w1128 stop-if-true
              n356 = Index Array(array=w1135, index=w1132) -> (element=w1136:string)
              n357 = xnode "Match Regular Expression"("input string"=w1136, "regular expression"=w1133) -> ("whole match"=w1134:string)  [unwired: 4 in, 4 out]
              n358 = Equal?(x=w1134, y=w1133) -> (x = y?=w1130:bool)
              n359 = Equal?(x=w1131, y=w1132) -> (x = y?=w1129:bool)
              n360 = Or(x=w1130, y=w1129) -> (x .or. y?=w1128:bool)
            }
            n361 = local write "Index 3"(w1045) -> ()
            n362 = Search 1D Array(1D array=w1091, element="Mobility (cm^2/Vs):") -> (index of element=w1096:i32)  [unwired: 1 in]
            n363 = Increment(x=w1096) -> (x+1=w1095:i32)
            n364 = Index Array(array=w1091, index=w1095) -> (element=w1093:string)
            n365 = Fract/Exp String To Number(string=w1093) -> (number=w1092:dbl)  [unwired: 3 in, 1 out]
            n366 = local write "Recorded Mobility"(w1092) -> ()
            n367 = Build Path(base path=w1043, name or relative path="ROI") -> (appended path=w1042:path)
            n368 = Path To String(path=w1043) -> (string=w1099:string)
            n369 = local read "No Image"() -> (w1053:path)
            n370 = Build Path(base path=w1042, name or relative path=w1045) -> (appended path=w1051:path)
            n371 = invoke on="Image Out" class="ImageControl" method="Clear ROI"(error in=w1046) -> (error out=w1050:errorcluster)  [unwired: 2 in, 2 out]
            n372 = Index Array(array=w1101, index=w1100) -> (element=w1056:string)
            n373 = Empty String/Path?(string/path=w1056) -> (empty?=w1057:bool)
            n374 = Concatenate Strings(w1099, "\\", w1056) -> (w1098:string)
            n375 = String To Path(string=w1098) -> (path=w1055:path)
            n376 = Select(t=w1053, s=w1057, f=w1055) -> (s? t:f=w1054:path)
            n377 = call "Vision Acquisition3"("Image Path"=w1054) -> ("Image Out"=w1102:T2)  [unwired: 25 in, 1 out]
            n378 = local write "Image File"(w1054) -> ()
            n379 = local write "Image Out 2"(w1102) -> ()
            n380 = local write "Image Out"(w1102) -> ()
            n381 = local write "Image Name"(w1056) -> ()
            n382 = call <vilib>:"Check if File or Folder Exists.vi"("error in (no error)"=w1050, "path"=w1051) -> ("file or folder exists?"=w1048:bool, "dup path"=w1049:path)  [unwired: 7 in, 1 out]
            n383 = invoke on="Image Out" class="ImageControl" method="Clear ROI"() -> ()  [unwired: 3 in, 3 out]
            n384 = case shown="True" w1048 {
              tunnel: w1049 -> [_ w1123]
              frame False {
              }
              frame True {
                n385 = Read from Text File(file (use dialog)=w1123) -> (text=w1127:string)  [unwired: 3 in, 3 out]
                n386 = property on="Image Out" class="ImageControl"() -> ("ROI"=w1124:T7)  [unwired: 2 in, 2 out]
                n387 = Unflatten From String(type=w1124, binary string=w1127) -> (value=w1125:T7, error out=w1126:errorcluster)  [unwired: 3 in, 1 out]
                n388 = property on="Image Out" class="ImageControl"(error in=w1126, "ROI"=w1125) -> ()  [unwired: 1 in, 2 out]
              }
            }
          }
          event "Up Button": Mouse Down {
            w1319 = 0
            n389 = event-data() -> ()  [unwired: 1 in, 5 out]
            n390 = local read "NumPts"() -> (w1290:dbl)
            n391 = local read "Row Start"() -> (w1289:dbl)
            n392 = local read "Data File"() -> (w1315:path)
            n393 = local read "NumPts 2"() -> (w1284:dbl)
            n394 = property on="Image Out" class="ImageControl"() -> (error out=w1248:errorcluster, "Image Center Position"=w1252:cluster{"X":u32, "Y":u32})  [unwired: 2 in, 1 out]
            n395 = Strip Path(path=w1315) -> (stripped path=w1314:path, name=w1335:string)
            n396 = local write "Data Folder"(w1314) -> ()
            n397 = List Folder(path=w1314) -> (filenames=w1325:string[], error out=w1258:errorcluster)  [unwired: 3 in, 2 out]
            n398 = Path To String(path=w1314) -> (string=w1336:string)
            n399 = Search 1D Array(1D array=w1325, element=w1335) -> (index of element=w1327:i32)  [unwired: 1 in]
            n400 = Equal To 0?(x=w1327) -> (x = 0?=w1328:bool)
            n401 = Unbundle(w1252) -> ("X"=w1250:u32)  [unwired: 1 out]
            n402 = Bundle("X"=w1250, 0) -> (w1251:cluster{"X":u32, i32})  [unwired: 1 in]
            n403 = property on="Image Out" class="ImageControl"(error in=w1248, "Image Center Position"=w1251) -> ()  [unwired: 1 in, 2 out]
            n404 = Array Size(array=w1325) -> (size(s)=w1324:i32)
            n405 = case shown="True" w1328 {
              tunnel: w1327 -> [w1463 _]
              tunnel: [w1462 w1464] -> w1326
              tunnel: w1324 -> [_ w1465]
              frame False {
                n406 = Decrement(x=w1463) -> (x-1=w1462:i32)
              }
              frame True {
                n407 = Decrement(x=w1465) -> (x-1=w1464:i32)
              }
            }
            n408 = Index Array(array=w1325, index=w1326) -> (element=w1329:string)
            n409 = local write "Data Name"(w1329) -> ()
            n410 = Concatenate Strings(w1336, "\\", w1329) -> (w1334:string)
            n411 = String To Path(string=w1334) -> (path=w1291:path)
            n412 = call "sub_thresh_swing_subvi.vi"("Path"=w1291, "NumPts"=w1284, "Row Start"=w1289) -> ("Index"=w1283:dbl, "XY Graph"=w1279:cluster{dbl[], dbl[]}[], "Sub Threshold Swing"=w1292:dbl)  [unwired: 8 in, 2 out]
            n413 = Decimate 1D Array(w1279) -> (w1282:cluster{dbl[], dbl[]}[])  [unwired: 1 out]
            n414 = Array To Cluster(array=w1282) -> (cluster=w1280:T5)
            n415 = Unbundle(w1280) -> ("[0]"=w1281:cluster{dbl[], dbl[]})  [unwired: 8 out]
            n416 = Unbundle(w1281) -> (w1278:dbl[], w1277:dbl[])
            n417 = Array Subset(array=w1278, index=w1283, length=w1284) -> (w1286:dbl[])
            n418 = Array Subset(array=w1277, index=w1283, length=w1284) -> (w1285:dbl[])
            n419 = local write "S.T.S."(w1292) -> ()
            n420 = local write "Array 8"(w1286) -> ()
            n421 = local write "Array 7"(w1285) -> ()
            n422 = call "mobility_subvi.vi"("Path"=w1291, "NumPts"=w1290, "Row Start"=w1289) -> ("Dielectric (d)"=w1294:dbl, "Index"=w1296:dbl, "XY Graph"=w1302:cluster{dbl[], dbl[]}[], "Length"=w1293:dbl, "Vt"=w1295:dbl, "Width"=w1270:dbl, "Table Control"=w1332:string[][], "Table Control 2"=w1331:string[][], "Recorded"=w1274:T6, "Mobility"=w1330:dbl)  [unwired: 2 in, 1 out]
            n423 = local write "Dielectric (d)"(w1294) -> ()
            n424 = local write "New Dielectric"(w1294) -> ()
            n425 = local write "New Length"(w1293) -> ()
            n426 = local write "New Width"(w1270) -> ()
            n427 = local write "Table Control"(w1332) -> ()
            n428 = Decimate 1D Array(w1302) -> (w1303:cluster{dbl[], dbl[]}[])  [unwired: 1 out]
            n429 = local write "XY Graph 2"(w1279) -> ()
            n430 = Array To Cluster(array=w1303) -> (cluster=w1305:T5)
            n431 = local write "XY Graph"(w1302) -> ()
            n432 = local write "Index 2"(w1283) -> ()
            n433 = local write "Table Control 2"(w1331) -> ()
            n434 = local write "Mobility"(w1330) -> ()
            n435 = local write "Length"(w1293) -> ()
            n436 = Unbundle(w1305) -> ("[0]"=w1304:cluster{dbl[], dbl[]})  [unwired: 8 out]
            n437 = Unbundle(w1304) -> (w1288:dbl[], w1287:dbl[])
            n438 = local write "Threshold V"(w1295) -> ()
            n439 = local write "Width"(w1270) -> ()
            n440 = Unbundle(w1274) -> ("Vt"=w1276:dbl, "STS"=w1275:dbl, "On/Off"=w1273:dbl)  [unwired: 4 out]
            n441 = Array Subset(array=w1288, index=w1296, length=w1290) -> (w1301:dbl[])
            n442 = Array Subset(array=w1287, index=w1296, length=w1290) -> (w1300:dbl[])
            n443 = local write "STS recorded"(w1275) -> ()
            n444 = local write "Data File"(w1291) -> ()
            n445 = local write "Index"(w1296) -> ()
            n446 = local write "Vt recorded"(w1276) -> ()
            n447 = local write "On/Off"(w1273) -> ()
            n448 = local write "Array 2"(w1300) -> ()
            n449 = local write "Array"(w1301) -> ()
            n450 = local read "Image Folder"() -> (w1262:path)
            n451 = local write "Slide"(w1296) -> ()
            n452 = List Folder(path=w1262, error in=w1258) -> (filenames=w1313:string[], error out=w1257:errorcluster)  [unwired: 2 in, 2 out]
            n453 = call-poly <vilib>:"Read From Spreadsheet File.vi"("file path (dialog if empty)"=w1291) -> ("all rows"=w1321:string[][])  [unwired: 6 in, 4 out]
            n454 = Array Size(array=w1321) -> (size(s)=w1320:i32[])
            n455 = Index Array(array=w1320, index=w1319) -> (element=w1298:i32)
            n456 = Subtract(x=w1298, y=20) -> (x-y=w1297:i32)
            n457 = property on="Slide" class="Slide (strict)"("Scale.Maximum"=w1297) -> ()  [unwired: 2 in, 2 out]
            n458 = Array Subset(array=w1321, index (row)=w1319, index (col)=w1319, length (col)=3) -> (w1322:string[][])  [unwired: 1 in]
            n459 = Reshape Array(w1322, w1298) -> (w1308:string[])
            n460 = Search 1D Array(1D array=w1308, element="Mobility (cm^2/Vs):") -> (index of element=w1311:i32)  [unwired: 1 in]
            n461 = Increment(x=w1311) -> (x+1=w1310:i32)
            n462 = Index Array(array=w1308, index=w1310) -> (element=w1307:string)
            n463 = Fract/Exp String To Number(string=w1307) -> (number=w1306:dbl)  [unwired: 3 in, 1 out]
            n464 = local write "Recorded Mobility"(w1306) -> ()
            n465 = Search 1D Array(1D array=w1308, element="Index:") -> (index of element=w1316:i32)  [unwired: 1 in]
            n466 = Increment(x=w1316) -> (x+1=w1317:i32)
            n467 = Index Array(array=w1308, index=w1317) -> (element=w1254:string)
            n468 = while {
              tunnel: w1313 -> [w1349]
              tunnel: w1254 -> [w1347]
              tunnel: [w1346] -> w1312
              tunnel: w1298 -> [w1345]
              i -> [w1346]
              stop <- w1342 stop-if-true
              n469 = Index Array(array=w1349, index=w1346) -> (element=w1350:string)
              n470 = xnode "Match Regular Expression"("input string"=w1350, "regular expression"=w1347) -> ("whole match"=w1348:string)  [unwired: 4 in, 4 out]
              n471 = Equal?(x=w1348, y=w1347) -> (x = y?=w1344:bool)
              n472 = Equal?(x=w1345, y=w1346) -> (x = y?=w1343:bool)
              n473 = Or(x=w1344, y=w1343) -> (x .or. y?=w1342:bool)
            }
            n474 = local write "Index 3"(w1254) -> ()
            n475 = Build Path(base path=w1262, name or relative path="ROI") -> (appended path=w1255:path)
            n476 = Build Path(base path=w1255, name or relative path=w1254) -> (appended path=w1253:path)
            n477 = invoke on="Image Out" class="ImageControl" method="Clear ROI"(error in=w1257) -> (error out=w1261:errorcluster)  [unwired: 2 in, 2 out]
            n478 = call <vilib>:"Check if File or Folder Exists.vi"("error in (no error)"=w1261, "path"=w1253) -> ("file or folder exists?"=w1259:bool, "dup path"=w1260:path)  [unwired: 7 in, 1 out]
            n479 = local read "No Image"() -> (w1271:path)
            n480 = Index Array(array=w1313, index=w1312) -> (element=w1264:string)
            n481 = Build Path(base path=w1262, name or relative path=w1264) -> (appended path=w1263:path)
            n482 = local write "Image Name"(w1264) -> ()
            n483 = Empty String/Path?(string/path=w1264) -> (empty?=w1272:bool)
            n484 = case shown="True" w1259 {
              tunnel: w1260 -> [_ w1337]
              frame False {
              }
              frame True {
                n485 = Read from Text File(file (use dialog)=w1337) -> (text=w1341:string)  [unwired: 3 in, 3 out]
                n486 = property on="Image Out" class="ImageControl"() -> ("ROI"=w1338:T7)  [unwired: 2 in, 2 out]
                n487 = Unflatten From String(type=w1338, binary string=w1341) -> (value=w1339:T7, error out=w1340:errorcluster)  [unwired: 3 in, 1 out]
                n488 = property on="Image Out" class="ImageControl"(error in=w1340, "ROI"=w1339) -> ()  [unwired: 1 in, 2 out]
              }
            }
            n489 = Select(t=w1271, s=w1272, f=w1263) -> (s? t:f=w1265:path)
            n490 = call "Vision Acquisition5"("Image Path"=w1265) -> ("Image Out"=w1269:T2)  [unwired: 25 in, 1 out]
            n491 = local write "Image File"(w1265) -> ()
            n492 = local write "Image Out 2"(w1269) -> ()
            n493 = local write "Image Out"(w1269) -> ()
            n494 = call <vilib>:"Get File Extension.vi"("file"=w1265) -> ("lowercase file extension"=w1267:string)  [unwired: 7 in, 3 out]
            n495 = local write "String"(w1267) -> ()
            n496 = Search 1D Array(1D array=string[] ["bmp", "jpeg", "png", "jpg", "gif"], element=w1267) -> (index of element=w1266:i32)  [unwired: 1 in]
            n497 = Less Than 0?(x=w1266) -> ()  [unwired: 1 out]
          }
          event "Save Changes? 3": Mouse Down {
            n498 = event-data() -> ()  [unwired: 1 in, 7 out]
            n499 = local read "Image Folder"() -> (w1466:path)
            n500 = Build Path(base path=w1466, name or relative path="ROI") -> (appended path=w1473:path)
            n501 = call <vilib>:"Check if File or Folder Exists.vi"("path"=w1473) -> ("file or folder exists?"=w1475:bool, "dup path"=w1472:path)  [unwired: 8 in, 1 out]
            n502 = case shown="False" w1475 {
              tunnel: w1472 -> [w1477 w1478]
              tunnel: [w1476 w1478] -> w1467
              frame False {
                n503 = Create Folder(path (use dialog)=w1477) -> (created path=w1476:path)  [unwired: 2 in, 2 out]
              }
              frame True {
              }
            }
            n504 = property on="Image Out" class="ImageControl"() -> ("ROI"=w1471:T7)  [unwired: 2 in, 2 out]
            n505 = local read "Index 3"() -> (w1469:string)
            n506 = Flatten To String(anything=w1471) -> (data string=w1470:string)  [unwired: 3 in, 2 out]
            n507 = Build Path(base path=w1467, name or relative path=w1469) -> (appended path=w1468:path)
            n508 = Write to Text File(file (use dialog)=w1468, text=w1470) -> ()  [unwired: 2 in, 3 out]
          }
          event "Next Button": Mouse Down {
            n509 = event-data() -> ()  [unwired: 1 in, 5 out]
            n510 = local read "XY Graph"() -> (w1491:cluster{dbl[], dbl[]}[])
            n511 = local read "NumPts"() -> (w1492:dbl)
            n512 = local read "Index"() -> (w1493:dbl)
            n513 = Decimate 1D Array(w1491) -> (w1487:cluster{dbl[], dbl[]}[], w1486:cluster{dbl[], dbl[]}[])
            n514 = Array To Cluster(array=w1487) -> (cluster=w1497:T5)
            n515 = Unbundle(w1497) -> ("[0]"=w1496:cluster{dbl[], dbl[]})  [unwired: 8 out]
            n516 = Increment(x=w1493) -> (x+1=w1488:dbl)
            n517 = Unbundle(w1496) -> (w1495:dbl[], w1494:dbl[])
            n518 = Array Subset(array=w1495, index=w1488, length=w1492) -> (w1484:dbl[])
            n519 = local write "Index"(w1488) -> ()
            n520 = Array Subset(array=w1494, index=w1488, length=w1492) -> (w1483:dbl[])
            n521 = Bundle(w1484, w1483) -> (w1490:cluster{dbl[], dbl[]})  [unwired: 1 in]
            n522 = Build Array (concatenate)(w1487, w1486, w1490) -> (w1489:cluster{dbl[], dbl[]}[])
            n523 = local write "XY Graph"(w1489) -> ()
            n524 = local read "New Dielectric"() -> (w1482:dbl)
            n525 = local write "Array 2"(w1483) -> ()
            n526 = local read "New Length"() -> (w1481:dbl)
            n527 = local write "Array"(w1484) -> ()
            n528 = local read "New Width"() -> (w1480:dbl)
            n529 = call "mob_calc_subvi.vi"("Width"=w1480, "Length"=w1481, "Dielectric (d)"=w1482, "Array 2"=w1483, "Array"=w1484) -> ("Vt"=w1479:dbl, "Mobility"=w1485:dbl)  [unwired: 5 in]
            n530 = local write "New Mobility"(w1485) -> ()
            n531 = local write "New Vt"(w1479) -> ()
          }
          event "Next Button 2": Mouse Down {
            n532 = event-data() -> ()  [unwired: 1 in, 7 out]
            n533 = local read "XY Graph 2"() -> (w1506:cluster{dbl[], dbl[]}[])
            n534 = local read "Index 2"() -> (w1508:dbl)
            n535 = local read "NumPts 2"() -> (w1507:dbl)
            n536 = Decimate 1D Array(w1506) -> (w1502:cluster{dbl[], dbl[]}[], w1501:cluster{dbl[], dbl[]}[])
            n537 = Array To Cluster(array=w1502) -> (cluster=w1512:T5)
            n538 = Unbundle(w1512) -> ("[0]"=w1511:cluster{dbl[], dbl[]})  [unwired: 8 out]
            n539 = Increment(x=w1508) -> (x+1=w1503:dbl)
            n540 = Unbundle(w1511) -> (w1510:dbl[], w1509:dbl[])
            n541 = local write "Index 2"(w1503) -> ()
            n542 = Array Subset(array=w1510, index=w1503, length=w1507) -> (w1499:dbl[])
            n543 = Array Subset(array=w1509, index=w1503, length=w1507) -> (w1498:dbl[])
            n544 = Bundle(w1499, w1498) -> (w1505:cluster{dbl[], dbl[]})  [unwired: 1 in]
            n545 = Build Array (concatenate)(w1502, w1501, w1505) -> (w1504:cluster{dbl[], dbl[]}[])
            n546 = local write "XY Graph 2"(w1504) -> ()
            n547 = local write "Array 8"(w1499) -> ()
            n548 = call "sts_calc_subvi.vi"("Array 2"=w1499, "Array"=w1498) -> ("STS"=w1500:dbl)  [unwired: 9 in]
            n549 = local write "Array 7"(w1498) -> ()
            n550 = local write "New S.T.S."(w1500) -> ()
          }
          event "Previous Button 2": Mouse Down {
            n551 = event-data() -> ()  [unwired: 1 in, 7 out]
            n552 = local read "XY Graph 2"() -> (w1522:cluster{dbl[], dbl[]}[])
            n553 = local read "NumPts 2"() -> (w1523:dbl)
            n554 = local read "Index 2"() -> (w1515:dbl)
            n555 = Decimate 1D Array(w1522) -> (w1519:cluster{dbl[], dbl[]}[], w1518:cluster{dbl[], dbl[]}[])
            n556 = Array To Cluster(array=w1519) -> (cluster=w1527:T5)
            n557 = Unbundle(w1527) -> ("[0]"=w1526:cluster{dbl[], dbl[]})  [unwired: 8 out]
            n558 = Decrement(x=w1515) -> (x-1=w1516:dbl)
            n559 = Unbundle(w1526) -> (w1525:dbl[], w1524:dbl[])
            n560 = local write "Index 2"(w1516) -> ()
            n561 = Array Subset(array=w1525, index=w1516, length=w1523) -> (w1513:dbl[])
            n562 = Array Subset(array=w1524, index=w1516, length=w1523) -> (w1514:dbl[])
            n563 = Bundle(w1513, w1514) -> (w1521:cluster{dbl[], dbl[]})  [unwired: 1 in]
            n564 = Build Array (concatenate)(w1519, w1518, w1521) -> (w1520:cluster{dbl[], dbl[]}[])
            n565 = local write "XY Graph 2"(w1520) -> ()
            n566 = local write "Array 7"(w1514) -> ()
            n567 = call "sts_calc_subvi.vi"("Array 2"=w1513, "Array"=w1514) -> ("STS"=w1517:dbl)  [unwired: 9 in]
            n568 = local write "Array 8"(w1513) -> ()
            n569 = local write "New S.T.S."(w1517) -> ()
          }
          event "Previous Button": Mouse Down {
            n570 = event-data() -> ()  [unwired: 1 in, 5 out]
            n571 = local read "XY Graph"() -> (w1541:cluster{dbl[], dbl[]}[])
            n572 = Decimate 1D Array(w1541) -> (w1538:cluster{dbl[], dbl[]}[], w1537:cluster{dbl[], dbl[]}[])
            n573 = local read "NumPts"() -> (w1542:dbl)
            n574 = local read "Index"() -> (w1536:dbl)
            n575 = Array To Cluster(array=w1538) -> (cluster=w1546:T5)
            n576 = Unbundle(w1546) -> ("[0]"=w1545:cluster{dbl[], dbl[]})  [unwired: 8 out]
            n577 = Decrement(x=w1536) -> (x-1=w1535:dbl)
            n578 = Unbundle(w1545) -> (w1544:dbl[], w1543:dbl[])
            n579 = local read "New Dielectric"() -> (w1529:dbl)
            n580 = Array Subset(array=w1544, index=w1535, length=w1542) -> (w1534:dbl[])
            n581 = Array Subset(array=w1543, index=w1535, length=w1542) -> (w1533:dbl[])
            n582 = local write "Index"(w1535) -> ()
            n583 = Bundle(w1534, w1533) -> (w1540:cluster{dbl[], dbl[]})  [unwired: 1 in]
            n584 = Build Array (concatenate)(w1538, w1537, w1540) -> (w1539:cluster{dbl[], dbl[]}[])
            n585 = local write "XY Graph"(w1539) -> ()
            n586 = local read "New Length"() -> (w1530:dbl)
            n587 = local write "Array 2"(w1533) -> ()
            n588 = local read "New Width"() -> (w1531:dbl)
            n589 = call "mob_calc_subvi.vi"("Width"=w1531, "Length"=w1530, "Dielectric (d)"=w1529, "Array 2"=w1533, "Array"=w1534) -> ("Vt"=w1528:dbl, "Mobility"=w1532:dbl)  [unwired: 5 in]
            n590 = local write "New Mobility"(w1532) -> ()
            n591 = local write "Array"(w1534) -> ()
            n592 = local write "New Vt"(w1528) -> ()
          }
          event "Slide": Value Change {
            n593 = event-data() -> ()  [unwired: 1 in, 5 out]
            n594 = local read "XY Graph"() -> (w1559:cluster{dbl[], dbl[]}[])
            n595 = local read "Slide"() -> (w1548:dbl)
            n596 = Decimate 1D Array(w1559) -> (w1556:cluster{dbl[], dbl[]}[], w1555:cluster{dbl[], dbl[]}[])
            n597 = local read "NumPts"() -> (w1560:dbl)
            n598 = Array To Cluster(array=w1556) -> (cluster=w1564:T5)
            n599 = Unbundle(w1564) -> ("[0]"=w1563:cluster{dbl[], dbl[]})  [unwired: 8 out]
            n600 = Unbundle(w1563) -> (w1562:dbl[], w1561:dbl[])
            n601 = local read "New Dielectric"() -> (w1549:dbl)
            n602 = Array Subset(array=w1562, index=w1548, length=w1560) -> (w1554:dbl[])
            n603 = Array Subset(array=w1561, index=w1548, length=w1560) -> (w1553:dbl[])
            n604 = local write "Index"(w1548) -> ()
            n605 = Bundle(w1554, w1553) -> (w1558:cluster{dbl[], dbl[]})  [unwired: 1 in]
            n606 = Build Array (concatenate)(w1556, w1555, w1558) -> (w1557:cluster{dbl[], dbl[]}[])
            n607 = local write "XY Graph"(w1557) -> ()
            n608 = local read "New Length"() -> (w1550:dbl)
            n609 = local write "Array 2"(w1553) -> ()
            n610 = local read "New Width"() -> (w1551:dbl)
            n611 = call "mob_calc_subvi.vi"("Width"=w1551, "Length"=w1550, "Dielectric (d)"=w1549, "Array 2"=w1553, "Array"=w1554) -> ("Vt"=w1547:dbl, "Mobility"=w1552:dbl)  [unwired: 5 in]
            n612 = local write "New Mobility"(w1552) -> ()
            n613 = local write "Array"(w1554) -> ()
            n614 = local write "New Vt"(w1547) -> ()
          }
          event "Slide 2": Value Change {
            n615 = event-data() -> ()  [unwired: 1 in, 5 out]
            n616 = local read "XY Graph 2"() -> (w1573:cluster{dbl[], dbl[]}[])
            n617 = local read "Slide 2"() -> (w1568:dbl)
            n618 = Decimate 1D Array(w1573) -> (w1570:cluster{dbl[], dbl[]}[], w1569:cluster{dbl[], dbl[]}[])
            n619 = local read "NumPts 2"() -> (w1574:dbl)
            n620 = Array To Cluster(array=w1570) -> (cluster=w1578:T5)
            n621 = Unbundle(w1578) -> ("[0]"=w1577:cluster{dbl[], dbl[]})  [unwired: 8 out]
            n622 = Unbundle(w1577) -> (w1576:dbl[], w1575:dbl[])
            n623 = Array Subset(array=w1576, index=w1568, length=w1574) -> (w1566:dbl[])
            n624 = Array Subset(array=w1575, index=w1568, length=w1574) -> (w1565:dbl[])
            n625 = local write "Index 2"(w1568) -> ()
            n626 = Bundle(w1566, w1565) -> (w1572:cluster{dbl[], dbl[]})  [unwired: 1 in]
            n627 = Build Array (concatenate)(w1570, w1569, w1572) -> (w1571:cluster{dbl[], dbl[]}[])
            n628 = local write "XY Graph 2"(w1571) -> ()
            n629 = local write "Array 7"(w1565) -> ()
            n630 = local write "Array 8"(w1566) -> ()
            n631 = call "sts_calc_subvi.vi"("Array 2"=w1566, "Array"=w1565) -> ("STS"=w1567:dbl)  [unwired: 9 in]
            n632 = local write "New S.T.S."(w1567) -> ()
          }
          event "Save Changes?": Mouse Down {
            n633 = event-data() -> ()  [unwired: 1 in, 5 out]
            n634 = flat-sequence {
              tunnel: [w1606] -> w1584
              tunnel: [w1605] -> w1582
              tunnel: [w1605] -> w1581
              tunnel: [w1588] -> w1579
              tunnel: w1584 -> [w1714]
              tunnel: [w1715] -> w1583
              tunnel: w1582 -> [w1715]
              tunnel: w1581 -> [w1713]
              tunnel: [w1711] -> w1580
              tunnel: w1579 -> [w1711]
              tunnel: w1583 -> [w1720]
              tunnel: w1580 -> [w1719]
              frame #0 {
                w1593 = -1
                w1586 = "S.T.S. (V/decade):"
                w1587 = "Threshold V (V):"
                (unwired) 3
                w1591 = 1
                n635 = local read "Data File"() -> (w1606:path)
                n636 = local read "New Dielectric"() -> (w1629:dbl)
                n637 = local read "New Width"() -> (w1619:dbl)
                n638 = local read "New Length"() -> (w1617:dbl)
                n639 = local read "New Mobility"() -> (w1628:dbl)
                n640 = flat-sequence {
                  tunnel: [w1642] -> w1585
                  tunnel: w1585 -> [w1659]
                  frame #0 {
                    # "Makes Empty File for Transformer Data"
                    n641 = local read "Data Folder"() -> (w1631:path)
                    n642 = Build Path(base path=w1631, name or relative path="Stats") -> (appended path=w1633:path)
                    n643 = call <vilib>:"Check if File or Folder Exists.vi"("path"=w1633) -> ("file or folder exists?"=w1634:bool, "dup path"=w1635:path)  [unwired: 8 in, 1 out]
                    n644 = case shown="False" w1634 {
                      tunnel: [w1639 w1641] -> w1636
                      tunnel: w1635 -> [w1640 w1641]
                      frame False {
                        n645 = Create Folder(path (use dialog)=w1640) -> (created path=w1639:path)  [unwired: 2 in, 2 out]
                      }
                      frame True {
                      }
                    }
                    n646 = Build Path(base path=w1636, name or relative path="Tranformer Data.txt") -> (appended path=w1638:path)
                    n647 = call-poly <vilib>:"Write To Spreadsheet File.vi"("append to file? (new file:F)"=TRUE, "file path (dialog if empty)"=w1638) -> ()  [unwired: 6 in, 1 out]
                  }
                  frame #1 {
                    # "Adds Headers if they don't exist"
                    n648 = Concatenate Strings("Stats\\", "Tranformer Data.txt") -> (w1649:string)
                    n649 = local read "Data Folder"() -> (w1648:path)
                    n650 = Build Path(base path=w1648, name or relative path=w1649) -> (appended path=w1642:path)
                    n651 = call-poly <vilib>:"Read From Spreadsheet File.vi"("file path (dialog if empty)"=w1642) -> ("first row"=w1647:string[])  [unwired: 6 in, 4 out]
                    n652 = Search 1D Array(1D array=w1647, element="DeviceID") -> (index of element=w1645:i32)  [unwired: 1 in]
                    n653 = Equal?(x=w1645, y=0) -> (x = y?=w1643:bool)
                    n654 = case shown="False" w1643 {
                      tunnel: w1642 -> [w1653 _]
                      frame False {
                        n655 = local read "Transformer \nHeaders"() -> (w1652:string[])
                        n656 = call-poly <vilib>:"Write To Spreadsheet File.vi"("1D data"=w1652, "file path (dialog if empty)"=w1653) -> ()  [unwired: 6 in, 1 out]
                      }
                      frame True {
                      }
                    }
                  }
                  frame #2 {
                    # "Adds current device if it doesn't exist"
                    n657 = local read "Current \nRecord"() -> (w1658:string[])
                    n658 = Index Array(array=w1658, index=0) -> (element=w1657:string)
                    n659 = Concatenate Strings("Stats\\", "Tranformer Data.txt") -> (w1662:string)
                    n660 = local read "Data Folder"() -> (w1661:path)
                    n661 = local write "Current Device ID"(w1657) -> ()
                    n662 = local read "Current Device ID"() -> (w1667:string)
                    n663 = Build Path(base path=w1661, name or relative path=w1662) -> (appended path=w1660:path)
                    n664 = call-poly <vilib>:"Read From Spreadsheet File.vi"("file path (dialog if empty)"=w1660) -> ("all rows"=w1654:string[][])  [unwired: 6 in, 4 out]
                    n665 = Index Array(array=w1654, index (col)=0) -> (element=w1655:string[])  [unwired: 1 in]
                    n666 = Search 1D Array(1D array=w1655, element=w1667) -> (index of element=w1656:i32)  [unwired: 1 in]
                    n667 = Equal?(x=w1656, y=-1) -> (x = y?=w1669:bool)
                    n668 = case shown="False" w1669 {
                      tunnel: w1659 -> [w1672 w1683]
                      tunnel: w1656 -> [w1675 _]
                      tunnel: w1654 -> [w1676 _]
                      frame False {
                        n669 = local read "Current \nRecord"() -> (w1674:string[])
                        n670 = Replace Array Subset(array=w1676, new element=w1674, index (row)=w1675) -> (w1673:string[][])  [unwired: 1 in]
                        n671 = flat-sequence {
                          tunnel: w1672 -> [w1677]
                          tunnel: w1673 -> [w1678]
                          tunnel: [w1678] -> w1671
                          tunnel: [w1677] -> w1670
                          tunnel: w1671 -> [w1680]
                          tunnel: w1670 -> [w1679]
                          frame #0 {
                            n672 = Delete(path (use dialog)=w1677) -> ()  [unwired: 4 in, 3 out]
                          }
                          frame #1 {
                            n673 = call-poly <vilib>:"Write To Spreadsheet File.vi"("append to file? (new file:F)"=TRUE, "2D data"=w1680, "file path (dialog if empty)"=w1679) -> ()  [unwired: 5 in, 1 out]
                          }
                        }
                      }
                      frame True {
                        n674 = local read "Current \nRecord"() -> (w1682:string[])
                        n675 = call-poly <vilib>:"Write To Spreadsheet File.vi"("append to file? (new file:F)"=TRUE, "1D data"=w1682, "file path (dialog if empty)"=w1683) -> ()  [unwired: 5 in, 1 out]
                      }
                    }
                  }
                }
                n676 = call-poly <vilib>:"Read From Spreadsheet File.vi"("file path (dialog if empty)"=w1606) -> ("all rows"=w1598:string[][])  [unwired: 6 in, 4 out]
                n677 = Number To Fractional String(number=w1617) -> (F-format string=w1609:string)  [unwired: 3 in]
                n678 = Replace Array Subset(array=w1598, new element=w1609, index (row)=12, index (col)=w1591) -> (w1613:string[][])
                n679 = Number To Fractional String(number=w1619) -> (F-format string=w1620:string)  [unwired: 3 in]
                n680 = Replace Array Subset(array=w1613, new element=w1620, index (row)=13, index (col)=w1591) -> (w1615:string[][])
                n681 = Number To Fractional String(number=w1628) -> (F-format string=w1607:string)  [unwired: 3 in]
                n682 = Number To Fractional String(number=w1629) -> (F-format string=w1608:string)  [unwired: 3 in]
                n683 = Number To Decimal String(number=w1617) -> (decimal integer string=w1616:string)  [unwired: 1 in]
                n684 = Strip Path(path=w1606) -> (stripped path=w1627:path)  [unwired: 1 out]
                n685 = local read "Index 3"() -> (w1622:string)
                n686 = Replace Array Subset(array=w1615, new element=w1607, index (row)=15, index (col)=w1591) -> (w1614:string[][])
                n687 = Number To Decimal String(number=w1619) -> (decimal integer string=w1618:string)  [unwired: 1 in]
                n688 = Path To String(path=w1627) -> (string=w1625:string)
                n689 = Replace Array Subset(array=w1614, new element=w1608, index (row)=7, index (col)=w1591) -> (w1590:string[][])
                n690 = call "Build Text"("Index"=w1622, "Length"=w1616, "Width"=w1618) -> ("Result"=w1623:string)  [unwired: 11 in, 1 out]
                n691 = Concatenate Strings(w1625, "\\", w1623) -> (w1624:string)
                n692 = String To Path(string=w1624) -> (path=w1605:path)
                n693 = Array Size(array=w1598) -> (size(s)=w1600:i32[])
                n694 = Index Array(array=w1600, index=0) -> (element=w1599:i32)
                n695 = Array Subset(array=w1598, index (row)=0, index (col)=0) -> (w1604:string[][])  [unwired: 2 in]
                n696 = Reshape Array(w1604, w1599) -> (w1592:string[])
                n697 = Search 1D Array(1D array=w1592, element=w1587) -> (index of element=w1596:i32)  [unwired: 1 in]
                n698 = Search 1D Array(1D array=w1592, element=w1586) -> (index of element=w1597:i32)  [unwired: 1 in]
                n699 = Equal?(x=w1596, y=w1593) -> (x = y?=w1594:bool)
                n700 = Equal?(x=w1597, y=w1593) -> (x = y?=w1595:bool)
                n701 = case shown="True" w1594 {
                  tunnel: w1596 -> [_ _]
                  tunnel: w1590 -> [w1701 w1709]
                  tunnel: [w1700 w1708] -> w1589
                  tunnel: w1587 -> [_ w1707]
                  frame False {
                    n702 = local read "New Vt"() -> (w1703:dbl)
                    n703 = Number To Fractional String(number=w1703) -> (F-format string=w1699:string)  [unwired: 3 in]
                    n704 = Replace Array Subset(array=w1701, new element=w1699, index (row)=17, index (col)=1) -> (w1700:string[][])
                  }
                  frame True {
                    n705 = local read "New Vt"() -> (w1710:dbl)
                    n706 = Number To Fractional String(number=w1710) -> (F-format string=w1706:string)  [unwired: 3 in]
                    n707 = Build Array(w1707, w1706) -> (w1705:string[])
                    n708 = Insert Into Array(array=w1709, index (row)=17, new element=w1705) -> (w1708:string[][])  [unwired: 1 in]
                  }
                }
                n709 = case shown="True" w1595 {
                  tunnel: w1597 -> [_ _]
                  tunnel: w1589 -> [w1688 w1696]
                  tunnel: [w1687 w1695] -> w1588
                  tunnel: w1586 -> [_ w1693]
                  frame False {
                    n710 = local read "New S.T.S."() -> (w1690:dbl)
                    n711 = Number To Fractional String(number=w1690) -> (F-format string=w1686:string)  [unwired: 3 in]
                    n712 = Replace Array Subset(array=w1688, new element=w1686, index (row)=18, index (col)=1) -> (w1687:string[][])
                  }
                  frame True {
                    n713 = local read "New S.T.S."() -> (w1697:dbl)
                    n714 = Number To Fractional String(number=w1697) -> (F-format string=w1694:string)  [unwired: 3 in]
                    n715 = Build Array(w1693, w1694) -> (w1692:string[])
                    n716 = Insert Into Array(array=w1696, index (row)=18, new element=w1692) -> (w1695:string[][])  [unwired: 1 in]
                  }
                }
              }
              frame #1 {
                n717 = Equal?(x=w1714, y=w1713) -> (x = y?=w1712:bool)
                n718 = case shown="False" w1712 {
                  tunnel: w1714 -> [w1718 _]
                  tunnel: w1713 -> [w1717 _]
                  frame False {
                    n719 = Move(source path=w1718, 9:TRUE, 10:w1717) -> ()  [unwired: 2 in, 3 out]
                  }
                  frame True {
                  }
                }
              }
              frame #2 {
                n720 = local write "Data File"(w1720) -> ()
                n721 = call-poly <vilib>:"Write To Spreadsheet File.vi"("2D data"=w1719, "file path (dialog if empty)"=w1720) -> ()  [unwired: 6 in, 1 out]
              }
            }
          }
          event "Save Changes? 2": Mouse Down {
            n722 = event-data() -> ()  [unwired: 1 in, 5 out]
            n723 = stacked-sequence {
              seq-local: [w1797 _ _ _ _] -> [_ w1850 _ _ _]
              seq-local: [w1796 _ _ _ _] -> [_ w1851 _ _ _]
              seq-local: [w1796 _ _ _ _] -> [_ w1849 _ _ _]
              seq-local: [w1779 _ _ _ _] -> [_ w1847 _ _ _]
              seq-local: [_ w1851 _ _ _] -> [_ _ w1856 _ _]
              seq-local: [_ w1847 _ _ _] -> [_ _ w1855 _ _]
              frame #0 {
                w1784 = -1
                w1777 = "S.T.S. (V/decade):"
                w1778 = "Threshold V (V):"
                (unwired) 3
                w1782 = 1
                n724 = local read "Data File"() -> (w1797:path)
                n725 = local read "New Width"() -> (w1810:dbl)
                n726 = local read "New Dielectric"() -> (w1820:dbl)
                n727 = local read "New Length"() -> (w1808:dbl)
                n728 = local read "New Mobility"() -> (w1819:dbl)
                n729 = call-poly <vilib>:"Read From Spreadsheet File.vi"("file path (dialog if empty)"=w1797) -> ("all rows"=w1789:string[][])  [unwired: 6 in, 4 out]
                n730 = Number To Fractional String(number=w1808) -> (F-format string=w1800:string)  [unwired: 3 in]
                n731 = Replace Array Subset(array=w1789, new element=w1800, index (row)=12, index (col)=w1782) -> (w1804:string[][])
                n732 = Number To Fractional String(number=w1810) -> (F-format string=w1811:string)  [unwired: 3 in]
                n733 = Replace Array Subset(array=w1804, new element=w1811, index (row)=13, index (col)=w1782) -> (w1806:string[][])
                n734 = Number To Fractional String(number=w1819) -> (F-format string=w1798:string)  [unwired: 3 in]
                n735 = Number To Fractional String(number=w1820) -> (F-format string=w1799:string)  [unwired: 3 in]
                n736 = Number To Decimal String(number=w1808) -> (decimal integer string=w1807:string)  [unwired: 1 in]
                n737 = Strip Path(path=w1797) -> (stripped path=w1818:path)  [unwired: 1 out]
                n738 = local read "Index 3"() -> (w1813:string)
                n739 = Replace Array Subset(array=w1806, new element=w1798, index (row)=15, index (col)=w1782) -> (w1805:string[][])
                n740 = Number To Decimal String(number=w1810) -> (decimal integer string=w1809:string)  [unwired: 1 in]
                n741 = Path To String(path=w1818) -> (string=w1816:string)
                n742 = Replace Array Subset(array=w1805, new element=w1799, index (row)=7, index (col)=w1782) -> (w1781:string[][])
                n743 = call "Build Text2"("Index"=w1813, "Length"=w1807, "Width"=w1809) -> ("Result"=w1814:string)  [unwired: 11 in, 1 out]
                n744 = Concatenate Strings(w1816, "\\", w1814) -> (w1815:string)
                n745 = String To Path(string=w1815) -> (path=w1796:path)
                n746 = Array Size(array=w1789) -> (size(s)=w1791:i32[])
                n747 = Index Array(array=w1791, index=0) -> (element=w1790:i32)
                n748 = Array Subset(array=w1789, index (row)=0, index (col)=0) -> (w1795:string[][])  [unwired: 2 in]
                n749 = Reshape Array(w1795, w1790) -> (w1783:string[])
                n750 = Search 1D Array(1D array=w1783, element=w1778) -> (index of element=w1787:i32)  [unwired: 1 in]
                n751 = Search 1D Array(1D array=w1783, element=w1777) -> (index of element=w1788:i32)  [unwired: 1 in]
                n752 = Equal?(x=w1787, y=w1784) -> (x = y?=w1785:bool)
                n753 = Equal?(x=w1788, y=w1784) -> (x = y?=w1786:bool)
                n754 = case shown="True" w1785 {
                  tunnel: w1787 -> [_ _]
                  tunnel: w1781 -> [w1837 w1845]
                  tunnel: [w1836 w1844] -> w1780
                  tunnel: w1778 -> [_ w1843]
                  frame False {
                    n755 = local read "New Vt"() -> (w1839:dbl)
                    n756 = Number To Fractional String(number=w1839) -> (F-format string=w1835:string)  [unwired: 3 in]
                    n757 = Replace Array Subset(array=w1837, new element=w1835, index (row)=17, index (col)=1) -> (w1836:string[][])
                  }
                  frame True {
                    n758 = local read "New Vt"() -> (w1846:dbl)
                    n759 = Number To Fractional String(number=w1846) -> (F-format string=w1842:string)  [unwired: 3 in]
                    n760 = Build Array(w1843, w1842) -> (w1841:string[])
                    n761 = Insert Into Array(array=w1845, index (row)=17, new element=w1841) -> (w1844:string[][])  [unwired: 1 in]
                  }
                }
                n762 = case shown="True" w1786 {
                  tunnel: w1788 -> [_ _]
                  tunnel: w1780 -> [w1824 w1832]
                  tunnel: [w1823 w1831] -> w1779
                  tunnel: w1777 -> [_ w1829]
                  frame False {
                    n763 = local read "New S.T.S."() -> (w1826:dbl)
                    n764 = Number To Fractional String(number=w1826) -> (F-format string=w1822:string)  [unwired: 3 in]
                    n765 = Replace Array Subset(array=w1824, new element=w1822, index (row)=18, index (col)=1) -> (w1823:string[][])
                  }
                  frame True {
                    n766 = local read "New S.T.S."() -> (w1833:dbl)
                    n767 = Number To Fractional String(number=w1833) -> (F-format string=w1830:string)  [unwired: 3 in]
                    n768 = Build Array(w1829, w1830) -> (w1828:string[])
                    n769 = Insert Into Array(array=w1832, index (row)=18, new element=w1828) -> (w1831:string[][])  [unwired: 1 in]
                  }
                }
              }
              frame #1 {
                n770 = Equal?(x=w1850, y=w1849) -> (x = y?=w1848:bool)
                n771 = case shown="False" w1848 {
                  tunnel: w1850 -> [w1854 _]
                  tunnel: w1849 -> [w1853 _]
                  frame False {
                    n772 = Move(source path=w1854, 9:TRUE, 10:w1853) -> ()  [unwired: 2 in, 3 out]
                  }
                  frame True {
                  }
                }
              }
              frame #2 {
                n773 = local write "Data File"(w1856) -> ()
                n774 = call-poly <vilib>:"Write To Spreadsheet File.vi"("2D data"=w1855, "file path (dialog if empty)"=w1856) -> ()  [unwired: 6 in, 1 out]
              }
              frame #3 {
                w1920 = 0
                n775 = local read "NumPts 2"() -> (w1879:dbl)
                n776 = local read "NumPts"() -> (w1886:dbl)
                n777 = local read "Row Start"() -> (w1885:dbl)
                n778 = local read "Data File"() -> (w1925:path)
                n779 = property on="Image Out" class="ImageControl"() -> (error out=w1860:errorcluster, "Image Center Position"=w1864:cluster{"X":u32, "Y":u32})  [unwired: 2 in, 1 out]
                n780 = Strip Path(path=w1925) -> (stripped path=w1916:path, name=w1938:string)
                n781 = local write "Data Folder"(w1916) -> ()
                n782 = List Folder(path=w1916) -> (filenames=w1931:string[])  [unwired: 3 in, 3 out]
                n783 = Unbundle(w1864) -> ("X"=w1862:u32)  [unwired: 1 out]
                n784 = Array Size(array=w1931) -> (size(s)=w1926:i32)
                n785 = Path To String(path=w1916) -> (string=w1939:string)
                n786 = Search 1D Array(1D array=w1931, element=w1938) -> (index of element=w1928:i32)  [unwired: 1 in]
                n787 = Bundle("X"=w1862, 0) -> (w1863:cluster{"X":u32, i32})  [unwired: 1 in]
                n788 = Decrement(x=w1926) -> (x-1=w1929:i32)
                n789 = Equal?(x=w1928, y=w1929) -> (x = y?=w1930:bool)
                n790 = case shown="False" w1930 {
                  tunnel: w1928 -> [w2061 _]
                  tunnel: [w2060 0] -> w1927
                  frame False {
                    n791 = Increment(x=w2061) -> (x+1=w2060:i32)
                  }
                  frame True {
                  }
                }
                n792 = Index Array(array=w1931, index=w1927) -> (element=w1932:string)
                n793 = local write "Data Name"(w1932) -> ()
                n794 = Concatenate Strings(w1939, "\\", w1932) -> (w1937:string)
                n795 = property on="Image Out" class="ImageControl"(error in=w1860, "Image Center Position"=w1863) -> ()  [unwired: 1 in, 2 out]
                n796 = String To Path(string=w1937) -> (path=w1887:path)
                n797 = call "sub_thresh_swing_subvi.vi"("Path"=w1887, "NumPts"=w1879, "Row Start"=w1885) -> ("Index"=w1880:dbl, "XY Graph"=w1875:cluster{dbl[], dbl[]}[], "Sub Threshold Swing"=w1888:dbl)  [unwired: 8 in, 2 out]
                n798 = Decimate 1D Array(w1875) -> (w1878:cluster{dbl[], dbl[]}[])  [unwired: 1 out]
                n799 = Array To Cluster(array=w1878) -> (cluster=w1876:T5)
                n800 = Unbundle(w1876) -> ("[0]"=w1877:cluster{dbl[], dbl[]})  [unwired: 8 out]
                n801 = Unbundle(w1877) -> (w1874:dbl[], w1873:dbl[])
                n802 = local write "S.T.S."(w1888) -> ()
                n803 = local write "XY Graph 2"(w1875) -> ()
                n804 = local write "Index 2"(w1880) -> ()
                n805 = call "mobility_subvi.vi"("Path"=w1887, "NumPts"=w1886, "Row Start"=w1885) -> ("Dielectric (d)"=w1891:dbl, "Index"=w1896:dbl, "XY Graph"=w1899:cluster{dbl[], dbl[]}[], "Length"=w1889:dbl, "Vt"=w1892:dbl, "Width"=w1890:dbl, "Table Control"=w1935:string[][], "Table Control 2"=w1934:string[][], "Recorded"=w1872:T6, "Mobility"=w1933:dbl)  [unwired: 2 in, 1 out]
                n806 = local write "Dielectric (d)"(w1891) -> ()
                n807 = local write "Threshold V"(w1892) -> ()
                n808 = local write "New Dielectric"(w1891) -> ()
                n809 = Decimate 1D Array(w1899) -> (w1900:cluster{dbl[], dbl[]}[])  [unwired: 1 out]
                n810 = Array To Cluster(array=w1900) -> (cluster=w1902:T5)
                n811 = local write "Table Control"(w1935) -> ()
                n812 = Unbundle(w1902) -> ("[0]"=w1901:cluster{dbl[], dbl[]})  [unwired: 8 out]
                n813 = Unbundle(w1901) -> (w1882:dbl[], w1881:dbl[])
                n814 = local write "XY Graph"(w1899) -> ()
                n815 = local write "Table Control 2"(w1934) -> ()
                n816 = local write "Mobility"(w1933) -> ()
                n817 = Array Subset(array=w1882, index=w1896, length=w1886) -> (w1898:dbl[])
                n818 = Array Subset(array=w1881, index=w1896, length=w1886) -> (w1897:dbl[])
                n819 = local write "Width"(w1890) -> ()
                n820 = local write "Length"(w1889) -> ()
                n821 = local write "Array 2"(w1897) -> ()
                n822 = Unbundle(w1872) -> ("Vt"=w1871:dbl, "STS"=w1870:dbl, "On/Off"=w1869:dbl)  [unwired: 4 out]
                n823 = local write "On/Off"(w1869) -> ()
                n824 = local write "Array"(w1898) -> ()
                n825 = local write "Slide"(w1896) -> ()
                n826 = local write "Index"(w1896) -> ()
                n827 = local write "STS recorded"(w1870) -> ()
                n828 = local write "Vt recorded"(w1871) -> ()
                n829 = Array Subset(array=w1874, index=w1880, length=w1879) -> (w1884:dbl[])
                n830 = Array Subset(array=w1873, index=w1880, length=w1879) -> (w1883:dbl[])
                n831 = local write "New Width"(w1890) -> ()
                n832 = local write "Data File"(w1887) -> ()
                n833 = local write "New Length"(w1889) -> ()
                n834 = local write "Array 8"(w1884) -> ()
                n835 = local write "Array 7"(w1883) -> ()
                n836 = call-poly <vilib>:"Read From Spreadsheet File.vi"("file path (dialog if empty)"=w1887) -> ("all rows"=w1922:string[][])  [unwired: 6 in, 4 out]
                n837 = local read "Image Folder"() -> (w1910:path)
                n838 = Array Size(array=w1922) -> (size(s)=w1921:i32[])
                n839 = List Folder(path=w1910) -> (filenames=w1915:string[])  [unwired: 3 in, 3 out]
                n840 = Index Array(array=w1921, index=w1920) -> (element=w1894:i32)
                n841 = Subtract(x=w1894, y=20) -> (x-y=w1893:i32)
                n842 = property on="Slide" class="Slide (strict)"("Scale.Maximum"=w1893) -> ()  [unwired: 2 in, 2 out]
                n843 = Array Subset(array=w1922, index (row)=w1920, index (col)=w1920, length (col)=3) -> (w1923:string[][])  [unwired: 1 in]
                n844 = Reshape Array(w1923, w1894) -> (w1903:string[])
                n845 = Search 1D Array(1D array=w1903, element="Mobility (cm^2/Vs):") -> (index of element=w1908:i32)  [unwired: 1 in]
                n846 = Search 1D Array(1D array=w1903, element="Index:") -> (index of element=w1917:i32)  [unwired: 1 in]
                n847 = Increment(x=w1917) -> (x+1=w1918:i32)
                n848 = Index Array(array=w1903, index=w1918) -> (element=w1913:string)
                n849 = while {
                  tunnel: w1915 -> [w1947]
                  tunnel: w1913 -> [w1945]
                  tunnel: [w1944] -> _
                  tunnel: [w1944] -> w1914
                  tunnel: w1894 -> [w1943]
                  i -> [w1944]
                  stop <- w1940 stop-if-true
                  n850 = Index Array(array=w1947, index=w1944) -> (element=w1948:string)
                  n851 = xnode "Match Regular Expression"("input string"=w1948, "regular expression"=w1945) -> ("whole match"=w1946:string)  [unwired: 4 in, 4 out]
                  n852 = Equal?(x=w1946, y=w1945) -> (x = y?=w1942:bool)
                  n853 = Equal?(x=w1943, y=w1944) -> (x = y?=w1941:bool)
                  n854 = Or(x=w1942, y=w1941) -> (x .or. y?=w1940:bool)
                }
                n855 = local write "Index 3"(w1913) -> ()
                n856 = Increment(x=w1908) -> (x+1=w1907:i32)
                n857 = local read "No Image"() -> (w1865:path)
                n858 = Index Array(array=w1903, index=w1907) -> (element=w1905:string)
                n859 = Fract/Exp String To Number(string=w1905) -> (number=w1904:dbl)  [unwired: 3 in, 1 out]
                n860 = local write "Recorded Mobility"(w1904) -> ()
                n861 = Path To String(path=w1910) -> (string=w1912:string)
                n862 = local read "Image Out"() -> (w1857:T2)
                n863 = Index Array(array=w1915, index=w1914) -> (element=w1867:string)
                n864 = Empty String/Path?(string/path=w1867) -> (empty?=w1868:bool)
                n865 = Concatenate Strings(w1912, "\\", w1867) -> (w1911:string)
                n866 = local write "Image Name"(w1867) -> ()
                n867 = String To Path(string=w1911) -> (path=w1866:path)
                n868 = Select(t=w1865, s=w1868, f=w1866) -> (s? t:f=w1859:path)
                n869 = local write "Image File"(w1859) -> ()
                n870 = call "IMAQ ReadFile"("File Path"=w1859, "Image"=w1857) -> ("Image Out"=w1858:T2)  [unwired: 5 in, 4 out]
                n871 = local write "Image Out 2"(w1858) -> ()
                n872 = local write "Image Out"(w1858) -> ()
                n873 = invoke on="Image Out" class="ImageControl" method="Clear ROI"() -> ()  [unwired: 3 in, 3 out]
              }
              frame #4 {
                n874 = local read "Image Folder"() -> (w2063:path)
                n875 = Build Path(base path=w2063, name or relative path="ROI") -> (appended path=w2065:path)
                n876 = local read "Index 3"() -> (w2064:string)
                n877 = Build Path(base path=w2065, name or relative path=w2064) -> (appended path=w2070:path)
                n878 = invoke on="Image Out" class="ImageControl" method="Clear ROI"() -> (error out=w2069:errorcluster)  [unwired: 3 in, 2 out]
                n879 = call <vilib>:"Check if File or Folder Exists.vi"("error in (no error)"=w2069, "path"=w2070) -> ("file or folder exists?"=w2067:bool, "dup path"=w2068:path)  [unwired: 7 in, 1 out]
                n880 = case shown="True" w2067 {
                  tunnel: w2068 -> [_ w2071]
                  frame False {
                  }
                  frame True {
                    n881 = Read from Text File(file (use dialog)=w2071) -> (text=w2075:string)  [unwired: 3 in, 3 out]
                    n882 = property on="Image Out" class="ImageControl"() -> ("ROI"=w2072:T7)  [unwired: 2 in, 2 out]
                    n883 = Unflatten From String(type=w2072, binary string=w2075) -> (value=w2073:T7, error out=w2074:errorcluster)  [unwired: 3 in, 1 out]
                    n884 = property on="Image Out" class="ImageControl"(error in=w2074, "ROI"=w2073) -> ()  [unwired: 1 in, 2 out]
                  }
                }
              }
            }
            n885 = flat-sequence {
              tunnel: [w1734] -> w1721
              tunnel: w1721 -> [w1748]
              frame #0 {
                # "Makes Empty File for Transformer Data"
                n886 = local read "Data Folder"() -> (w1723:path)
                n887 = Build Path(base path=w1723, name or relative path="Stats") -> (appended path=w1725:path)
                n888 = call <vilib>:"Check if File or Folder Exists.vi"("path"=w1725) -> ("file or folder exists?"=w1726:bool, "dup path"=w1727:path)  [unwired: 8 in, 1 out]
                n889 = case shown="False" w1726 {
                  tunnel: [w1731 w1733] -> w1728
                  tunnel: w1727 -> [w1732 w1733]
                  frame False {
                    n890 = Create Folder(path (use dialog)=w1732) -> (created path=w1731:path)  [unwired: 2 in, 2 out]
                  }
                  frame True {
                  }
                }
                n891 = Build Path(base path=w1728, name or relative path="Tranformer Data.txt") -> (appended path=w1730:path)
                n892 = call-poly <vilib>:"Write To Spreadsheet File.vi"("append to file? (new file:F)"=TRUE, "file path (dialog if empty)"=w1730) -> ()  [unwired: 6 in, 1 out]
              }
              frame #1 {
                # "Adds Headers if they don't exist"
                n893 = Concatenate Strings("Stats\\", "Tranformer Data.txt") -> (w1741:string)
                n894 = local read "Data Folder"() -> (w1740:path)
                n895 = Build Path(base path=w1740, name or relative path=w1741) -> (appended path=w1734:path)
                n896 = call-poly <vilib>:"Read From Spreadsheet File.vi"("file path (dialog if empty)"=w1734) -> ("first row"=w1739:string[])  [unwired: 6 in, 4 out]
                n897 = Search 1D Array(1D array=w1739, element="DeviceID") -> (index of element=w1737:i32)  [unwired: 1 in]
                n898 = Equal?(x=w1737, y=0) -> (x = y?=w1735:bool)
                n899 = case shown="False" w1735 {
                  tunnel: w1734 -> [w1745 _]
                  frame False {
                    n900 = local read "Transformer \nHeaders"() -> (w1744:string[])
                    n901 = call-poly <vilib>:"Write To Spreadsheet File.vi"("1D data"=w1744, "file path (dialog if empty)"=w1745) -> ()  [unwired: 6 in, 1 out]
                  }
                  frame True {
                  }
                }
              }
              frame #2 {
                # "Adds current device if it doesn't exist"
                n902 = local read "Current \nRecord"() -> (w1751:string[])
                n903 = Index Array(array=w1751, index=0) -> (element=w1750:string)
                n904 = Concatenate Strings("Stats\\", "Tranformer Data.txt") -> (w1754:string)
                n905 = local read "Data Folder"() -> (w1753:path)
                n906 = local write "Current Device ID"(w1750) -> ()
                n907 = local read "Current Device ID"() -> (w1760:string)
                n908 = Build Path(base path=w1753, name or relative path=w1754) -> (appended path=w1752:path)
                n909 = call-poly <vilib>:"Read From Spreadsheet File.vi"("file path (dialog if empty)"=w1752) -> ("all rows"=w1747:string[][])  [unwired: 6 in, 4 out]
                n910 = Index Array(array=w1747, index (col)=0) -> (element=w1758:string[])  [unwired: 1 in]
                n911 = Search 1D Array(1D array=w1758, element=w1760) -> (index of element=w1746:i32)  [unwired: 1 in]
                n912 = Equal?(x=w1746, y=-1) -> (x = y?=w1749:bool)
                n913 = case shown="False" w1749 {
                  tunnel: w1748 -> [w1762 w1775]
                  tunnel: w1746 -> [w1767 _]
                  tunnel: w1747 -> [w1768 _]
                  frame False {
                    n914 = local read "Current \nRecord"() -> (w1766:string[])
                    n915 = Replace Array Subset(array=w1768, new element=w1766, index (row)=w1767) -> (w1763:string[][])  [unwired: 1 in]
                    n916 = flat-sequence {
                      tunnel: [w1769] -> _
                      tunnel: [w1770] -> _
                      tunnel: [w1770] -> w1765
                      tunnel: [w1769] -> w1764
                      tunnel: w1763 -> [w1770]
                      tunnel: w1762 -> [w1769]
                      tunnel: w1765 -> [w1772]
                      tunnel: w1764 -> [w1771]
                      frame #0 {
                        n917 = Delete(path (use dialog)=w1769) -> ()  [unwired: 4 in, 3 out]
                      }
                      frame #1 {
                        n918 = call-poly <vilib>:"Write To Spreadsheet File.vi"("append to file? (new file:F)"=TRUE, "2D data"=w1772, "file path (dialog if empty)"=w1771) -> ()  [unwired: 5 in, 1 out]
                      }
                    }
                  }
                  frame True {
                    n919 = local read "Current \nRecord"() -> (w1774:string[])
                    n920 = call-poly <vilib>:"Write To Spreadsheet File.vi"("append to file? (new file:F)"=TRUE, "1D data"=w1774, "file path (dialog if empty)"=w1775) -> ()  [unwired: 5 in, 1 out]
                  }
                }
              }
            }
          }
          event "Export": Mouse Down {
            n921 = event-data() -> ()  [unwired: 1 in, 7 out]
            n922 = call "OA_ConnectToOrigin.vi"() -> ("error out"=w2097:errorcluster, "Origin.IOApplication"=w2098:refnum<k7>)  [unwired: 8 in]
            n923 = local read "Data Folder"() -> (w2076:path)
            n924 = local read "Project"() -> (w2096:path)
            n925 = call "OA_Load.vi"("error in (no error)"=w2097, "Path"=w2096, "Origin.IOApplication"=w2098) -> ("error out"=w2089:errorcluster, "Origin.IOApplication"=w2090:refnum<k7>)  [unwired: 1 out]
            n926 = call "OAExecute.vi"("script"="document -m 3;", "Error IO"=w2089, "Origin.IOApplication"=w2090) -> ("Error IO Out"=w2087:errorcluster, "Origin.IOApplication"=w2088:refnum<k7>)  [unwired: 1 in, 1 out]
            n927 = Build Path(base path=w2076, name or relative path="Stats") -> (appended path=w2077:path)
            n928 = flat-sequence {
              tunnel: w2076 -> [w2118]
              tunnel: w2095 -> [w2117]
              tunnel: [w2107] -> w2100
              tunnel: [w2108] -> w2099
              tunnel: w2088 -> [w2112]
              tunnel: w2087 -> [w2111]
              tunnel: w2076 -> [w2134]
              tunnel: w2095 -> [w2133]
              tunnel: w2100 -> [w2129]
              tunnel: w2099 -> [w2130]
              tunnel: [w2124] -> w2094
              tunnel: [w2123] -> w2093
              tunnel: w2076 -> [w2145]
              tunnel: w2095 -> [w2144]
              tunnel: w2094 -> [w2140]
              tunnel: w2093 -> [w2139]
              tunnel: [w2138] -> w2092
              tunnel: [w2137] -> w2091
              tunnel: w2076 -> [w2160]
              tunnel: w2095 -> [w2159]
              tunnel: w2092 -> [w2154]
              tunnel: w2091 -> [w2153]
              tunnel: [w2151] -> w2085
              tunnel: [w2150] -> w2084
              frame #0 {
                n929 = call "Param_Analysis.vi"("error in (no error)"=w2111, "Folder 2"=w2118, "Parameter String"="Mobility (cm^2/Vs):", "Parameter Name"="Mobility", "Folder"=w2117) -> ("error out"=w2114:errorcluster, "Array 4"=w2104:string[], "Array 3"=w2113:string[][])  [unwired: 3 in, 1 out]
                n930 = call "Origin_Export.vi"("String 3"="[MobHistTab]Sheet1", "error in (no error)"=w2114, "Array"=w2113, "String 2"="[MOBvsLTable]Mobilities", "String"="pe_cd \"Mobility Chart\";", "Origin.IOApplication"=w2112, "Array 2"=w2104) -> ("reference out"=w2110:refnum<k7>, "error out"=w2109:errorcluster)  [unwired: 2 in, 1 out]
                n931 = call "OAExecute.vi"("script"="window -a MOBvsLTable;\nwindow -s TV;", "Error IO"=w2109, "Origin.IOApplication"=w2110) -> ("Error IO Out"=w2107:errorcluster, "Origin.IOApplication"=w2108:refnum<k7>)  [unwired: 1 in, 1 out]
              }
              frame #1 {
                n932 = call "Param_Analysis.vi"("error in (no error)"=w2129, "Folder 2"=w2134, "Parameter String"="On/Off Current:", "Parameter Name"="On_Off_Current", "Folder"=w2133) -> ("error out"=w2128:errorcluster, "Array 4"=w2122:string[], "Array 3"=w2125:string[][])  [unwired: 3 in, 1 out]
                n933 = call "Origin_Export.vi"("String 3"="[OnOffHistTab]Sheet1", "error in (no error)"=w2128, "Array"=w2125, "String 2"="[OnOffTable]On/Off Ratios", "String"="pe_cd \"OnOff vs L\";", "Origin.IOApplication"=w2130, "Array 2"=w2122) -> ("reference out"=w2124:refnum<k7>, "error out"=w2123:errorcluster)  [unwired: 2 in, 1 out]
              }
              frame #2 {
                n934 = call "Param_Analysis.vi"("Folder 2"=w2145, "Parameter String"="S.T.S. (V/decade):", "Parameter Name"="STS", "Folder"=w2144) -> ("Array 4"=w2136:string[], "Array 3"=w2141:string[][])  [unwired: 4 in, 2 out]
                n935 = call "Origin_Export.vi"("String 3"="[SHistTab]Sheet1", "error in (no error)"=w2139, "Array"=w2141, "String 2"="[STable]Threshold Swing", "String"="pe_cd \"Threshold Swing vs L\";", "Origin.IOApplication"=w2140, "Array 2"=w2136) -> ("reference out"=w2137:refnum<k7>, "error out"=w2138:errorcluster)  [unwired: 2 in, 1 out]
              }
              frame #3 {
                n936 = call "Param_Analysis.vi"("Folder 2"=w2160, "Parameter String"="Threshold V (V):", "Parameter Name"="Threshold_V", "Folder"=w2159) -> ("Array 4"=w2149:string[], "Array 3"=w2152:string[][])  [unwired: 4 in, 2 out]
                n937 = call "Origin_Export.vi"("String 3"="[VtHistTab]Sheet1", "error in (no error)"=w2154, "Array"=w2152, "String 2"="[VtTable]Threshold Voltages", "String"="pe_cd \"Threshold Voltage vs L\";", "Origin.IOApplication"=w2153, "Array 2"=w2149) -> ("reference out"=w2151:refnum<k7>, "error out"=w2150:errorcluster)  [unwired: 2 in, 1 out]
              }
            }
            n938 = call <vilib>:"Check if File or Folder Exists.vi"("path"=w2077) -> ("file or folder exists?"=w2102:bool, "dup path"=w2101:path)  [unwired: 8 in, 1 out]
            n939 = case shown="False" w2102 {
              tunnel: w2101 -> [w2162 w2163]
              tunnel: [w2161 w2163] -> w2095
              frame False {
                n940 = Create Folder(path (use dialog)=w2162) -> (created path=w2161:path)  [unwired: 2 in, 2 out]
              }
              frame True {
              }
            }
            n941 = call "File Dialog"("start path"=w2077) -> ("selected path"=w2080:path)  [unwired: 11 in, 3 out]
            n942 = Path To String(path=w2080) -> (string=w2079:string)
            n943 = call "OAExecute.vi"("script"="pe_cd /;\npe_cd \"Mobility Chart\"; ", "Error IO"=w2084, "Origin.IOApplication"=w2085) -> ("Error IO Out"=w2081:errorcluster, "Origin.IOApplication"=w2082:refnum<k7>)  [unwired: 1 in, 1 out]
            n944 = call "OASaveProject.vi"("path"=w2079, "Error IO"=w2081, "Origin.IOApplication"=w2082) -> ()  [unwired: 3 out]
          }
          event "Blank Button": Mouse Down {
            n945 = event-data() -> ()  [unwired: 1 in, 7 out]
            n946 = local read "Data File"() -> (w2171:path)
            n947 = Strip Path(path=w2171) -> (stripped path=w2167:path, name=w2169:string)
            n948 = Path To String(path=w2167) -> (string=w2166:string)
            n949 = Concatenate Strings(w2166, "\\", "X_", w2169) -> (w2165:string)
            n950 = String To Path(string=w2165) -> (path=w2164:path)
            n951 = Move(source path=w2171, 10:w2164) -> ()  [unwired: 3 in, 3 out]
            n952 = local write "Data File"(w2164) -> ()
          }
          event "Cancel Button": Mouse Down {
            (unwired) 6
            n953 = event-data() -> ()  [unwired: 1 in, 7 out]
            n954 = call "Simulate_Keyboard.vi"("Action"=2, "Virtual Key"=162) -> ()  [unwired: 7 in, 1 out]
          }
        }
        n955 = local read "New Length"() -> (w405:dbl)
        n956 = local read "New Width"() -> (w404:dbl)
        n957 = local read "Accel (RPM/s):"() -> (w432:dbl)
        n958 = local read "Sample #:"() -> (w424:dbl)
        n959 = local read "New Mobility"() -> (w434:dbl)
        n960 = local read "Method Recorded"() -> (w425:string)
        n961 = local read "# Drops:"() -> (w442:dbl)
        n962 = local read "Ramp (s):"() -> (w450:dbl)
        n963 = local read "Solvent Recorded"() -> (w400:string)
        n964 = local read "New S.T.S."() -> (w426:dbl)
        n965 = local read "Date Recorded"() -> (w421:string)
        n966 = local read "Time (s):"() -> (w437:dbl)
        n967 = local read "On/Off"() -> (w430:dbl)
        n968 = local read "New Vt"() -> (w428:dbl)
        n969 = local read "RPM:"() -> (w438:dbl)
        n970 = local read "Fabricator:"() -> (w446:string)
        n971 = Number To Decimal String(number=w442) -> (decimal integer string=w443:string)  [unwired: 1 in]
        n972 = Number To Decimal String(number=w424) -> (decimal integer string=w417:string)  [unwired: 1 in]
        n973 = call "DeviceID"("Sample"=w417, "Year"=w418, "Month"=w412, "Day"=w408, "Index"=w406) -> ("Result"=w423:string)  [unwired: 9 in, 1 out]
        n974 = Number To Decimal String(number=w405) -> (decimal integer string=w403:string)  [unwired: 1 in]
        n975 = Number To Decimal String(number=w404) -> (decimal integer string=w402:string)  [unwired: 1 in]
        n976 = Number To Decimal String(number=w441) -> (decimal integer string=w440:string)  [unwired: 1 in]
        n977 = Number To Decimal String(number=w396) -> (decimal integer string=w395:string)  [unwired: 1 in]
        n978 = Number To Decimal String(number=w445) -> (decimal integer string=w444:string)  [unwired: 1 in]
        n979 = Number To Decimal String(number=w399) -> (decimal integer string=w397:string)  [unwired: 1 in]
        n980 = Number To Decimal String(number=w438) -> (decimal integer string=w439:string)  [unwired: 1 in]
        n981 = Number To Fractional String(number=w432) -> (F-format string=w433:string)  [unwired: 3 in]
        n982 = Number To Decimal String(number=w437) -> (decimal integer string=w436:string)  [unwired: 1 in]
        n983 = Number To Fractional String(number=w434) -> (F-format string=w435:string)  [unwired: 3 in]
        n984 = Number To Fractional String(number=w430) -> (F-format string=w431:string)  [unwired: 3 in]
        n985 = Number To Fractional String(number=w428) -> (F-format string=w429:string)  [unwired: 3 in]
        n986 = Number To Fractional String(number=w426) -> (F-format string=w427:string)  [unwired: 3 in]
        n987 = Number To Decimal String(number=w450) -> (decimal integer string=w451:string)  [unwired: 1 in]
        n988 = property on="Image Out" class="ImageControl"() -> ("ROI"=w458:T7)  [unwired: 2 in, 2 out]
        n989 = local read "Image Out"() -> (w487:T2)
        n990 = Build Array(w423, w446, w425, w421, w417, w447, w448, w403, w402, w394, w398, w397, w400, w401, w440, w443, w453, w444, w395, w451, w439, w433, w436, w435, w431, w429, w427) -> (w449:string[])
        n991 = local write "Current \nRecord"(w449) -> ()
        n992 = property on="Image Out" class="ImageControl"() -> ("ZoomSingle"=w501:cluster{"X":sgl, "Y":sgl})  [unwired: 2 in, 2 out]
        n993 = property on="Image Out" class="ImageControl"() -> ("Bounds"=w502:T8)  [unwired: 2 in, 2 out]
        n994 = Unbundle By Name(w458) -> ("Contours"=w532:T9)
        n995 = call <vilib>:"Intialize Keyboard.vi"() -> ("device ID"=w513:refnum<k1>)  [unwired: 10 in, 1 out]
        n996 = property on="Image Out" class="ImageControl"() -> ("Image Center Position"=w508:cluster{"X":u32, "Y":u32})  [unwired: 2 in, 2 out]
        n997 = call "IMAQ Clear Overlay"("Image"=w487) -> ("Image Out"=w486:T2)  [unwired: 9 in, 1 out]
        n998 = call-poly <vilib>:"Acquire Input Data.vi"("device ID"=w513) -> ("keys pressed"=w512:T10)  [unwired: 16 in, 2 out]
        n999 = Initialize Array(0) -> (w530:i32[])  [unwired: 1 in]
        n1000 = local read "Magnification"() -> (w521:u16)
        n1001 = Unbundle(w502) -> ("Width"=w499:u32, "Height"=w498:u32)
        n1002 = Array Size(array=w532) -> (size(s)=w531:i32)
        n1003 = Unbundle(w501) -> ("X"=w476:sgl, "Y"=w500:sgl)
        n1004 = event shown="[2] \" Image Folder\": Value Change" {
          selector: _ -> [_ _ _ _ _ _ _]
          dyn-events: _ -> [_ _ _ _ _ _ _]
          timeout: 10 -> [_ _ _ _ _ _ _]
          event "Remove Button": Mouse Down {
            w546 = 0
            n1005 = property on="Image Out" class="ImageControl"() -> ("ROI"=w544:T7)  [unwired: 2 in, 2 out]
            n1006 = event-data() -> ()  [unwired: 1 in, 7 out]
            n1007 = Unbundle(w544) -> ("Global Rectangle"=w547:i32[], "Contours"=w549:T9)
            n1008 = Reverse 1D Array(array=w547) -> (reversed array=w548:i32[])
            n1009 = Reverse 1D Array(array=w549) -> (reversed array=w550:T9)
            n1010 = Delete From Array(array=w548, index=w546) -> (array with subset deleted=w551:i32[])  [unwired: 1 in, 1 out]
            n1011 = Delete From Array(array=w550, index=w546) -> (array with subset deleted=w552:T9)  [unwired: 1 in, 1 out]
            n1012 = Reverse 1D Array(array=w551) -> (reversed array=w553:i32[])
            n1013 = Reverse 1D Array(array=w552) -> (reversed array=w554:T9)
            n1014 = Bundle(w553, w554) -> (w545:T11)  [unwired: 1 in]
            n1015 = local write "ROI Descriptor out"(w544) -> ()
            n1016 = local write "ROI Descriptor"(w545) -> ()
            n1017 = property on="Image Out" class="ImageControl"("ROI"=w545) -> ()  [unwired: 2 in, 2 out]
          }
          event "Undo Button": Mouse Down {
            n1018 = event-data() -> ()  [unwired: 1 in, 7 out]
            n1019 = invoke on="Image Out" class="ImageControl" method="Clear ROI"() -> ()  [unwired: 3 in, 3 out]
          }
          event "Image Folder": Value Change {
            n1020 = event-data() -> ()  [unwired: 1 in, 5 out]
            n1021 = local read "Image File"() -> (w556:path)
            n1022 = call "Vision Acquisition"("Image Path"=w556) -> ("Image Out"=w555:T2)  [unwired: 25 in, 1 out]
            n1023 = local write "Image Out 2"(w555) -> ()
            n1024 = local write "Image Out"(w555) -> ()
            n1025 = invoke on="Image Out" class="ImageControl" method="Clear ROI"() -> ()  [unwired: 3 in, 3 out]
          }
          event "Zoom": Value Change {
            n1026 = event-data() -> ()  [unwired: 1 in, 5 out]
            n1027 = local read "Zoom"() -> (w557:i16)
            n1028 = Bundle("Zoom"=w557, "Zoom"=w557) -> (w558:cluster{"Zoom":i16, "Zoom":i16})  [unwired: 1 in]
            n1029 = property on="Image Out" class="ImageControl"("ZoomInteger"=w558) -> ()  [unwired: 2 in, 2 out]
          }
          event Timeout {
            n1030 = event-data() -> ()  [unwired: 1 in, 2 out]
          }
          event "Image Out": Mouse Enter {
            (unwired) 6
            n1031 = event-data() -> ()  [unwired: 1 in, 3 out]
            n1032 = call "Simulate_Keyboard.vi"("Action"=0, "Virtual Key"=162) -> ()  [unwired: 7 in, 1 out]
          }
          event "Image Out": Mouse Leave {
            n1033 = event-data() -> ()  [unwired: 1 in, 3 out]
            n1034 = flat-sequence {
              frame #0 {
                n1035 = Wait (ms)(milliseconds to wait=10) -> ()  [unwired: 1 out]
              }
              frame #1 {
                (unwired) 6
                n1036 = call "Simulate_Keyboard.vi"("Action"=2, "Virtual Key"=162) -> ()  [unwired: 7 in, 1 out]
              }
            }
          }
        }
        n1037 = Build Array(0.505025, 0.252522, 0.127742, 0.050345, 0.031129) -> (w522:dbl[])
        n1038 = Index Array(array=w512) -> (element=w516:T12)  [unwired: 1 in]
        n1039 = Divide(x=w499, y=w476) -> (x/y=w489:sgl)
        n1040 = Multiply(x=w489, y=0.5) -> (x*y=w495:dbl)
        n1041 = Divide(x=w498, y=w500) -> (x/y=w488:sgl)
        n1042 = Multiply(x=w488, y=0.5) -> (x*y=w494:dbl)
        n1043 = Array Subset(array=w522, index=w521, length=1) -> (w519:dbl[])
        n1044 = property on="Image Out" class="ImageControl"() -> ("ZoomInteger"=w511:cluster{"X":i32, "Y":i32})  [unwired: 2 in, 2 out]
        n1045 = Unbundle(w508) -> ("X"=w490:u32, "Y"=w491:u32)
        n1046 = Subtract(x=w491, y=w494) -> (x-y=w492:dbl)
        n1047 = Subtract(x=w490, y=w495) -> (x-y=w493:dbl)
        n1048 = Add(x=w493, y=w489) -> (x+y=w507:dbl)
        n1049 = Add(x=w492, y=w488) -> (x+y=w506:dbl)
        n1050 = To Double Precision Float(number=w519) -> (double precision float=w518:dbl[])
        n1051 = local write "ROI Descriptor"(w458) -> ()
        n1052 = Reciprocal(x=w476) -> (1/x=w475:sgl)
        n1053 = Unbundle(w511) -> ("X"=w510:i32)  [unwired: 1 out]
        n1054 = Multiply(x=w475, y=10) -> (x*y=w477:sgl)
        n1055 = case shown="\"EQUALS\"" w516 {
          tunnel: w490 -> [w565 w571 w575 w577 w581 w583 w585 w587 w589 w591 w593 w595 w597 w599 w601 w603 w605 w607 w609 w611 w613 w615 w617 w619 w621 w623 w625 w627 w629 w631 w633 w635 w637 w639 w641 w643 w645 w647 w649 w651 w653 w655 w657 w659 w661 w663 w665 w667 w669 w671 w673 w675 w677 w679 w681 w683 w685 w687 w689 w691 w693 w695 w697 w699 w701 w703 w705 w707 w709 w711 w713 w715 w717 w719 w721 w723 w725 w727 w729 w731 w733 w735 w737 w739 w741 w743 w745 w747 w749 w751 w753 w755 w757 w759 w761 w763 w765 w767 w769 w771 w773 w775 w777 w779 w781]
          tunnel: [w565 w570 w574 w577 w581 w583 w585 w587 w589 w591 w593 w595 w597 w599 w601 w603 w605 w607 w609 w611 w613 w615 w617 w619 w621 w623 w625 w627 w629 w631 w633 w635 w637 w639 w641 w643 w645 w647 w649 w651 w653 w655 w657 w659 w661 w663 w665 w667 w669 w671 w673 w675 w677 w679 w681 w683 w685 w687 w689 w691 w693 w695 w697 w699 w701 w703 w705 w707 w709 w711 w713 w715 w717 w719 w721 w723 w725 w727 w729 w731 w733 w735 w737 w739 w741 w743 w745 w747 w749 w751 w753 w755 w757 w759 w761 w763 w765 w767 w769 w771 w773 w775 w777 w779 w781] -> w515
          tunnel: w491 -> [w567 w569 w573 w579 w580 w582 w584 w586 w588 w590 w592 w594 w596 w598 w600 w602 w604 w606 w608 w610 w612 w614 w616 w618 w620 w622 w624 w626 w628 w630 w632 w634 w636 w638 w640 w642 w644 w646 w648 w650 w652 w654 w656 w658 w660 w662 w664 w666 w668 w670 w672 w674 w676 w678 w680 w682 w684 w686 w688 w690 w692 w694 w696 w698 w700 w702 w704 w706 w708 w710 w712 w714 w716 w718 w720 w722 w724 w726 w728 w730 w732 w734 w736 w738 w740 w742 w744 w746 w748 w750 w752 w754 w756 w758 w760 w762 w764 w766 w768 w770 w772 w774 w776 w778 w780]
          tunnel: [w566 w569 w573 w578 w580 w582 w584 w586 w588 w590 w592 w594 w596 w598 w600 w602 w604 w606 w608 w610 w612 w614 w616 w618 w620 w622 w624 w626 w628 w630 w632 w634 w636 w638 w640 w642 w644 w646 w648 w650 w652 w654 w656 w658 w660 w662 w664 w666 w668 w670 w672 w674 w676 w678 w680 w682 w684 w686 w688 w690 w692 w694 w696 w698 w700 w702 w704 w706 w708 w710 w712 w714 w716 w718 w720 w722 w724 w726 w728 w730 w732 w734 w736 w738 w740 w742 w744 w746 w748 w750 w752 w754 w756 w758 w760 w762 w764 w766 w768 w770 w772 w774 w776 w778 w780] -> w514
          tunnel: w477 -> [w564 w568 w572 w576 _ _ _ _ _ _ _ _ _ _ _ _ _ _ _ _ _ _ _ _ _ _ _ _ _ _ _ _ _ _ _ _ _ _ _ _ _ _ _ _ _ _ _ _ _ _ _ _ _ _ _ _ _ _ _ _ _ _ _ _ _ _ _ _ _ _ _ _ _ _ _ _ _ _ _ _ _ _ _ _ _ _ _ _ _ _ _ _ _ _ _ _ _ _ _ _ _ _ _ _ _]
          frame "DOWN" {
            n1056 = Add(x=w567, y=w564) -> (x+y=w566:sgl)
          }
          frame "LEFT" {
            n1057 = Subtract(x=w571, y=w568) -> (x-y=w570:sgl)
          }
          frame "RIGHT" {
            n1058 = Add(x=w575, y=w572) -> (x+y=w574:sgl)
          }
          frame "UP" {
            n1059 = Subtract(x=w579, y=w576) -> (x-y=w578:sgl)
          }
          frame "ENTER (num pad)" {
          }
          frame "' (quote)" {
          }
          frame "END" {
          }
          frame "EQUALS" {
          }
          frame "ESCAPE" {
          }
          frame "GRAVE (`)" {
          }
          frame "HOME" {
          }
          frame "INSERT" {
          }
          frame "LBRACKET" {
          }
          frame "LCONTROL" {
          }
          frame "L ALT" {
          }
          frame "LSHIFT" {
          }
          frame "LWIN" {
          }
          frame "MINUS" {
          }
          frame "MULTIPLY" {
          }
          frame "NEXT" {
          }
          frame "NUMLOCK" {
          }
          frame "NUMPAD_0" {
          }
          frame "NUMPAD_1" {
          }
          frame "NUMPAD_2" {
          }
          frame "NUMPAD_3" {
          }
          frame "NUMPAD_4" {
          }
          frame "NUMPAD_5" {
          }
          frame "NUMPAD_6" {
          }
          frame "NUMPAD_7" {
          }
          frame "NUMPAD_8" {
          }
          frame "NUMPAD_9" {
          }
          frame "PAUSE" {
          }
          frame "PERIOD" {
          }
          frame "PRIOR (PG UP)" {
          }
          frame "RBRACKET" {
          }
          frame "RCONTROL" {
          }
          frame "RETURN" {
          }
          frame "R ALT" {
          }
          frame "RSHIFT" {
          }
          frame "RWIN" {
          }
          frame "SCROLL" {
          }
          frame "SEMICOLON" {
          }
          frame "SLASH" {
          }
          frame "SPACE" {
          }
          frame "SUBTRACT" {
          }
          frame "TAB" {
          }
          frame "DIVIDE" {
          }
          frame "DELETE" {
          }
          frame "DECIMAL" {
          }
          frame "COMMA" {
          }
          frame "CAPITAL" {
          }
          frame "BACKSLASH" {
          }
          frame "BACK" {
          }
          frame "ADD" {
          }
          frame "F15" {
          }
          frame "F14" {
          }
          frame "F13" {
          }
          frame "F12" {
          }
          frame "F11" {
          }
          frame "F10" {
          }
          frame "F9" {
          }
          frame "F8" {
          }
          frame "F7" {
          }
          frame "F6" {
          }
          frame "F5" {
          }
          frame "F4" {
          }
          frame "F3" {
          }
          frame "F2" {
          }
          frame "F1" {
          }
          frame "Z" {
          }
          frame "Y" {
          }
          frame "X" {
          }
          frame "W" {
          }
          frame "V" {
          }
          frame "U" {
          }
          frame "T" {
          }
          frame "S" {
          }
          frame "R" {
          }
          frame "Q" {
          }
          frame "P" {
          }
          frame "O" {
          }
          frame "N" {
          }
          frame "M" {
          }
          frame "L" {
          }
          frame "K" {
          }
          frame "J" {
          }
          frame "I" {
          }
          frame "H" {
          }
          frame "G" {
          }
          frame "F" {
          }
          frame "E" {
          }
          frame "D" {
          }
          frame "C" {
          }
          frame "B" {
          }
          frame "A" {
          }
          frame "9" {
          }
          frame "8" {
          }
          frame "7" {
          }
          frame "6" {
          }
          frame "5" {
          }
          frame "4" {
          }
          frame "3" {
          }
          frame "2" {
          }
          frame "1" {
          }
          frame "0" {
          }
        }
        n1060 = Bundle(w493, w492, w507, w506, 0.0) -> (w505:cluster{dbl, dbl, dbl, dbl, dbl})  [unwired: 1 in]
        n1061 = Bundle("X"=w515, "Y"=w514) -> (w509:cluster{"X":sgl, "Y":sgl})  [unwired: 1 in]
        n1062 = Divide(x=20, y=w476) -> (x/y=w479:sgl)
        n1063 = local write "Zoom"(w510) -> ()
        n1064 = property on="Image Out" class="ImageControl"("Image Center Position"=w509) -> ()  [unwired: 2 in, 2 out]
        n1065 = call "IMAQ Convert Rectangle to ROI (Polygon)"("Rectangle"=w505) -> ("ROI Descriptor"=w503:T3)  [unwired: 7 in, 2 out]
        n1066 = Bundle("Application Font", w479, w483, w483, w483, w483, w483, TRUE, w481) -> (w485:T13)  [unwired: 1 in]
        n1067 = property on="Image Out 2" class="ImageControl"("ROI"=w503) -> ()  [unwired: 2 in, 2 out]
        n1068 = Bundle(w481, w485, w481, w481) -> (w484:T14)  [unwired: 1 in]
        n1069 = for {
          N: w531 -> [_]
          shift-right: [w804] -> _
          shift-left: w532 -> [w804]
          shift-right: [w802] -> w517
          shift-left: w530 -> [w801]
          tunnel: w518 -> [w800]
          shift-right: [w797] -> _
          shift-left: w486 -> [w799]
          tunnel: w484 -> [w792]
          i -> [w796]
          n1070 = Index Array(array=w804, index=w796) -> (element=w813:T15)
          n1071 = Unbundle(w813) -> ("Points"=w812:i32[])  [unwired: 2 out]
          n1072 = Array To Cluster(array=w812) -> (cluster=w811:T16)
          n1073 = Unbundle(w811) -> ("Points[0]"=w791:i32, "Points[1]"=w788:i32, "Points[2]"=w803:i32, "Points[3]"=w809:i32)  [unwired: 5 out]
          n1074 = Add(x=w791, y=10) -> (x+y=w789:i32)
          n1075 = Subtract(x=w788, y=w809) -> (x-y=w808:i32)
          n1076 = Subtract(x=w791, y=w803) -> (x-y=w810:i32)
          n1077 = Square(x=w808) -> (x^2=w806:i32)
          n1078 = Square(x=w810) -> (x^2=w807:i32)
          n1079 = Add(x=w807, y=w806) -> (x+y=w805:i32)
          n1080 = Square Root(x=w805) -> (sqrt(x)=w782:dbl)
          n1081 = Multiply(x=w782, y=0.5) -> (x*y=w785:dbl)
          n1082 = Add(x=w785, y=w788) -> (x+y=w787:dbl)
          n1083 = Bundle(w789, w787) -> (w798:cluster{i32, dbl})  [unwired: 1 in]
          n1084 = Multiply(x=w782, y=w800) -> (x*y=w795:dbl[])
          n1085 = Index Array(array=w795) -> (element=w794:dbl)  [unwired: 1 in]
          n1086 = Number To Fractional String(number=w794) -> (F-format string=w793:string)  [unwired: 3 in]
          n1087 = call "IMAQ Overlay Text"("BG Color (Transparent)"=u32 0, "Text Color (black)"=u32 16448250, "Font, Size & Style"=w792, "String"=w793, "Origin"=w798, "Image"=w799) -> ("Image Out"=w797:T2)  [unwired: 4 in, 1 out]
          n1088 = Build Array (concatenate)(w801, w795) -> (w802:dbl[])
          n1089 = local write "Numeric 3"(w782) -> ()
        }
        n1090 = Add Array Elements(numeric array=w517) -> (sum=w528:dbl)
        n1091 = local write "Distances"(w517) -> ()
        n1092 = local write "Total Width"(w528) -> ()
        n1093 = local read "Array 8"() -> (w463:dbl[])
        n1094 = local read "Array 7"() -> (w464:dbl[])
        n1095 = local read "Width"() -> (w459:dbl)
        n1096 = local read "New Dielectric"() -> (w471:dbl)
        n1097 = local read "Array 2"() -> (w467:dbl[])
        n1098 = local read "Manual"() -> (w457:bool)
        n1099 = local read "New Length"() -> (w469:dbl)
        n1100 = local read "Array"() -> (w468:dbl[])
        n1101 = call "sts_calc_subvi.vi"("Array 2"=w463, "Array"=w464) -> ("STS"=w465:dbl)  [unwired: 9 in]
        n1102 = local read "New Width"() -> (w472:dbl)
        n1103 = local write "New S.T.S."(w465) -> ()
        n1104 = call "mob_calc_subvi.vi"("Width"=w472, "Length"=w469, "Dielectric (d)"=w471, "Array 2"=w467, "Array"=w468) -> ("Vt"=w466:dbl, "Mobility"=w470:dbl)  [unwired: 5 in]
        n1105 = Not(x=w457) -> (.not. x?=w455:bool)
        n1106 = local write "New Vt"(w466) -> ()
        n1107 = local write "New Mobility"(w470) -> ()
        n1108 = local read "Total Width"() -> (w461:dbl)
        n1109 = Equal To 0?(x=w461) -> (x = 0?=w456:bool)
        n1110 = And(x=w456, y=w455) -> (x .and. y?=w454:bool)
        n1111 = case shown="True" w454 {
          tunnel: w459 -> [_ w542]
          frame False {
          }
          frame True {
            n1112 = local write "New Width"(w542) -> ()
          }
        }
        n1113 = Or(x=w456, y=w457) -> (x .or. y?=w460:bool)
        n1114 = case shown="False" w460 {
          tunnel: w461 -> [w543 _]
          frame False {
            n1115 = local write "New Width"(w543) -> ()
          }
          frame True {
          }
        }
      }
    }
  }
  n1116 = disable-structure shown="Disabled" {
    frame Disabled {
      n1117 = local read "Data Folder"() -> ()  [unwired: 1 out]
      n1118 = local read "Data Folder"() -> ()  [unwired: 1 out]
      n1119 = local read "Data Folder"() -> ()  [unwired: 1 out]
    }
    frame Enabled {
    }
  }
  n1120 = Build Array("DeviceID", "Fabricator", "Deposition", "Date", "Sample", "Row", "Column", "L (um)", "W (um)", "Material", "Treatment", "TC (mM)", "Solvent", "C (%)", "ST (C)", "Drops", "Wait (s)", "RT (F)", "RH (%)", "Ramp (s)", "RPM", "Accel (RPM/s)", "Time (s)", "Mobility", "On/Off", "Vt", "S.T.S") -> (→"Transformer \nHeaders":string[])
